vi "Process Mngr.vi"(0 "State In":T5, 1 "Mngr Action":T12, 2 "FP":T11, 7 "Cartridges":T4, 9 "Manual Input":dbl format="%#_13g", 11 "error in (no error)":errorcluster, 12 "Config":T1={"Syringe size"=0, "Syringe address"=0, "# of ports"=0, "Init String"="Z0N1R", "Full Stroke (cnts)"=0, "Model"=enum."XC", "TW Position"=0.0, "Load Position"=0.0, "Bottom Position"=0.0, "Station ID"="", "Default Protocol"=path "", "Dry Time(s)"=0.0, "Python Version"="", "NFC SN Array"=["21121521200223", "21121521200186", "21121521200213", "52541737200062"], "Timing"={"Checking pres and leak"=0.0, "Priming input lines"=0.0, "Rinsing syringe"=0.0, "Filling well X w/ X"=0.0, "Drain well X"=0.0, "Clearing wells and lines"=0.0, "Draining wells"=0.0, "Rinsing all wells"=0.0, "Testing for leaks/clogs"=0.0, "Rinsing wells"=0.0}, "Pressure Specs"={"Pressure max"=0.0, "Pressure min"=0.0, "Decay delta"=0.0, "Pressure time"=0.0, "Conf. R"=0.0, "LeakRateMax"=0.0}}) -> (6 "State Out":T5, 15 "error out":errorcluster)   [LabVIEW 2020]
uses:
  Process Mngr.ctl
  Main Refs.ctl
  Hardware/Tecan/Pump Config.ctl
  Timing Specs.ctl
  Vacuum Specs.ctl
  Cartridges.ctl
  Cartridge Status.ctl
  Commands.ctl
  Lib/Time/Wells.ctl
  Lib/Time/Bottles.ctl
  Process State.ctl
  Vacuum Test.ctl
  Wash Step.ctl
  Results.ctl
  Vacuum Output.ctl
  Cartridge #.ctl
  status update.ctl
  Cartridge Mngr.ctl
  Time elapsed.ctl
  Hardware/DAQ Mngr.ctl
  Hardware/Mot Stage Mngr.ctl
  Update Single Cart.ctl
  Hardware/Denkovi Mngr.ctl
  Hardware/Tricon Mngr.ctl
  Hardware/Tecan/Pump Control.ctl
  Pump Port.ctl
  Hardware/Tecan/Velocity Units.ctl
  Main Globals.vi
  Lib/Utilities.lvlib
panel:
  out "Reports":T6[](array[typedef])
  in  "Pressure Specs":T9
  out "Wash Array":T10[](array[typedef]) {"# of Rinses" max=10}
  # "Tecan Pump"
  # "Pressure"
  # "General"
  # "Timing"
  # "Protocol"
  # "Zaber"
  # "NFC Reader 1"
  # "NFC  Reader 2"
  # "NFC Reader 3"
  # "NFC Reader 4"
  # "Tecan Pump"
  # "Pressure"
  # "General"
  # "Timing"
  # "Protocol"
  # "Zaber"
  # "NFC Reader 1"
  # "NFC  Reader 2"
  # "NFC Reader 3"
  # "NFC Reader 4"
  # "System"
  # "Cartridge Utitlies"
  # "Wells"
  # "times"
  # "from"
  # "State Machine"
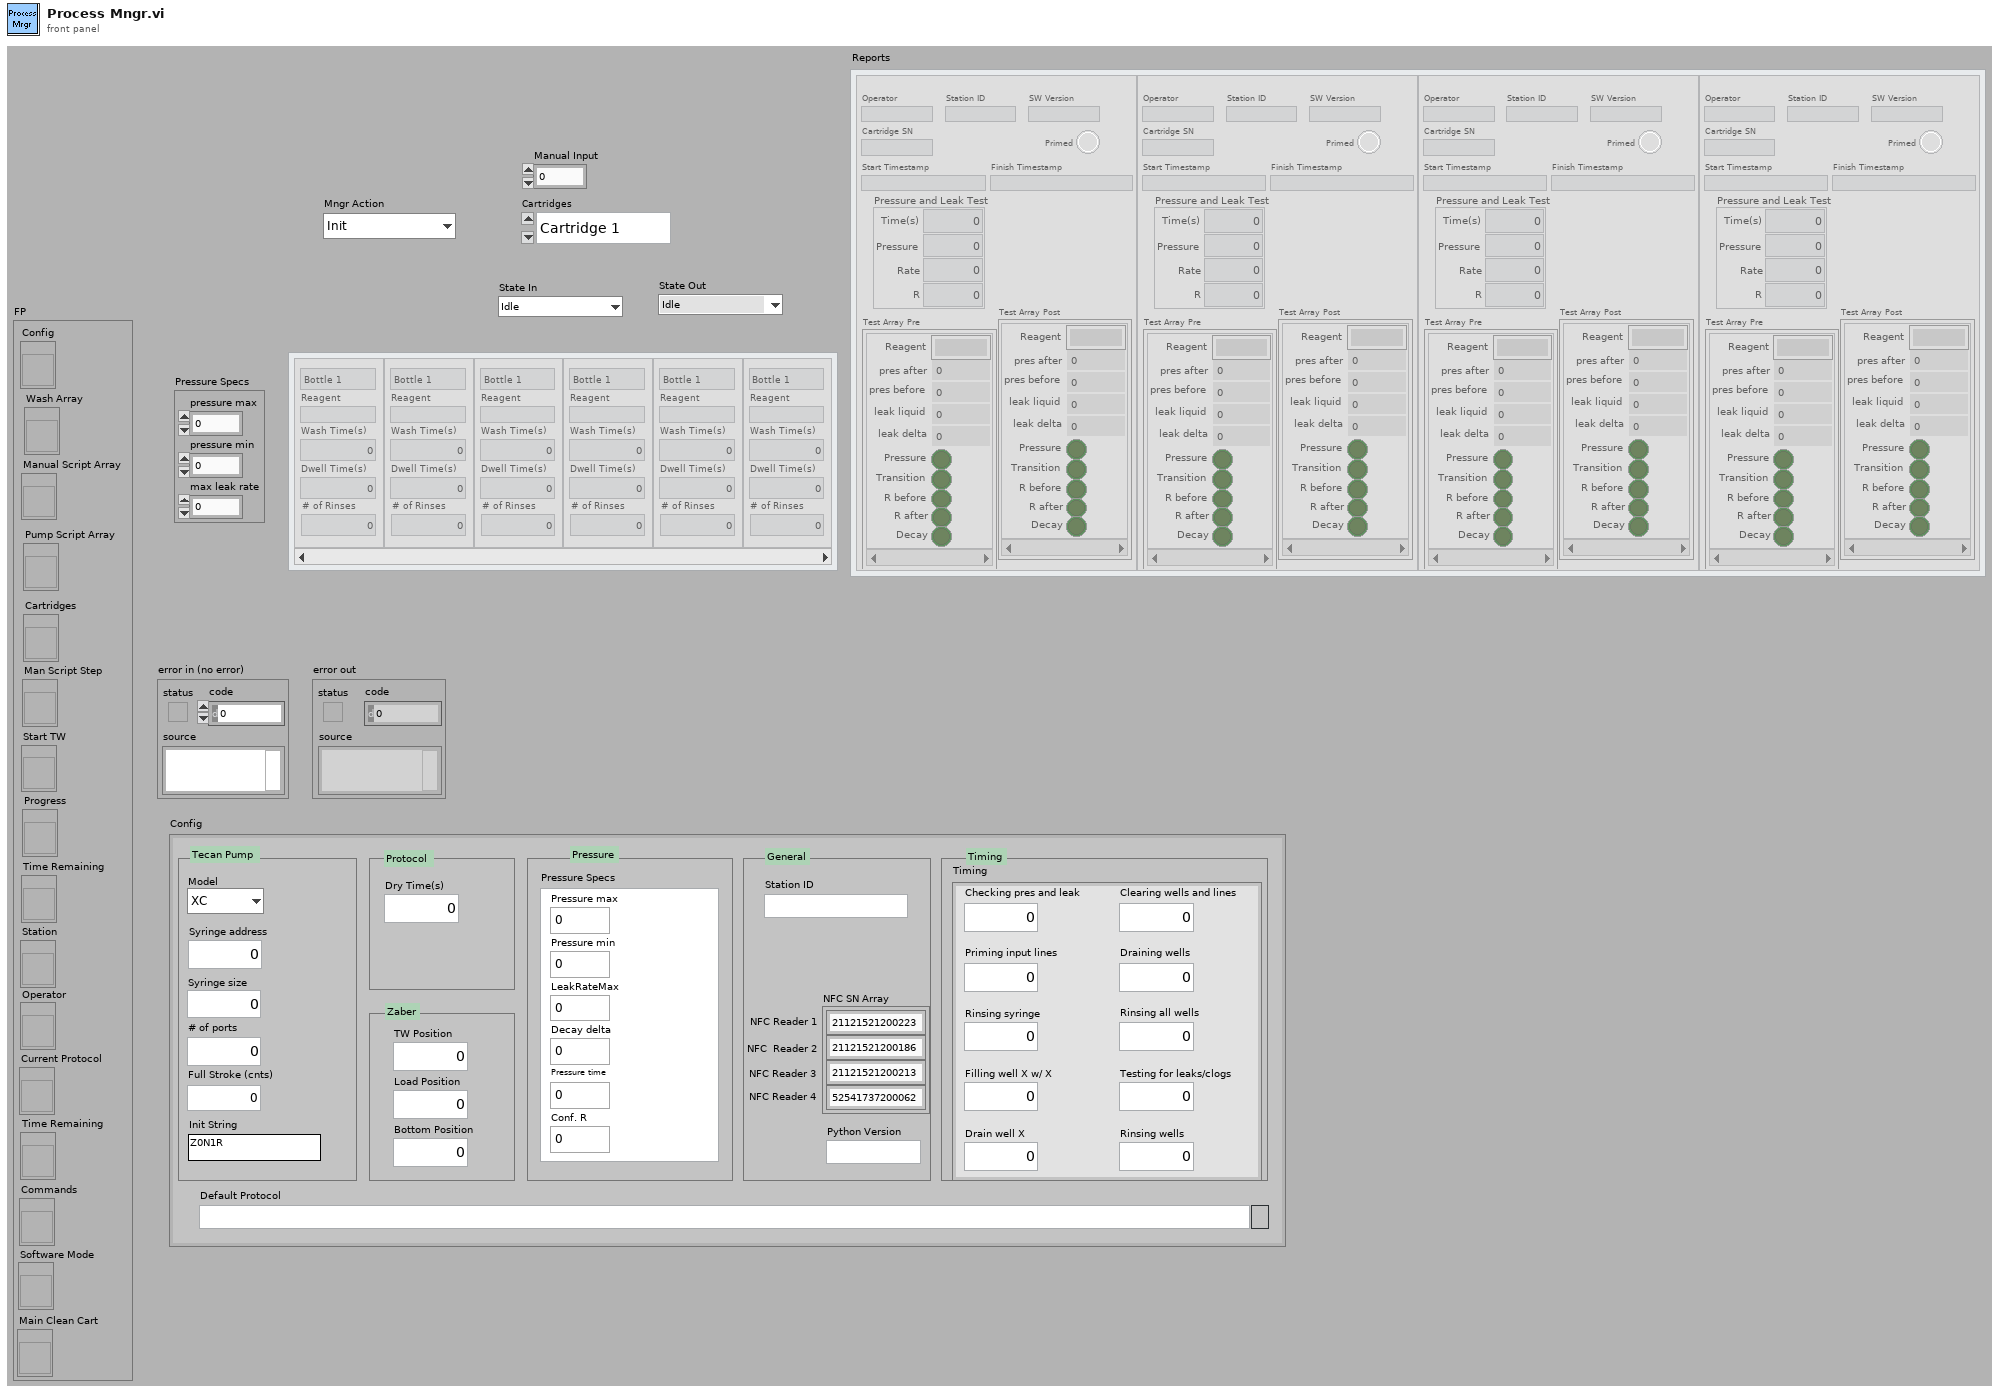
[diagram p1: front panel]
types:
  T1 = typedef "Pump Config.ctl" = cluster{"Syringe size":u32, "Syringe address":u32, "# of ports":u32, "Init String":string, "Full Stroke (cnts)":i32, "Model":enum16{"XC", "Centris"}, "TW Position":dbl, "Load Position":dbl, "Bottom Position":dbl, "Station ID":string, "Default Protocol":path, "Dry Time(s)":dbl, "Python Version":string, "NFC SN Array":string[], "Timing":T2, "Pressure Specs":T3}
  T2 = typedef "Timing Specs.ctl" = cluster{"Checking pres and leak":dbl, "Priming input lines":dbl, "Rinsing syringe":dbl, "Filling well X w/ X":dbl, "Drain well X":dbl, "Clearing wells and lines":dbl, "Draining wells":dbl, "Rinsing all wells":dbl, "Testing for leaks/clogs":dbl, "Rinsing wells":dbl}
  T3 = typedef "Vacuum Specs.ctl" = cluster{"Pressure max":dbl, "Pressure min":dbl, "Decay delta":dbl, "Pressure time":dbl, "Conf. R":dbl, "LeakRateMax":dbl}
  T4 = typedef "Cartridge #.ctl" = enum16{"Cartridge 1", "Cartridge 2", "Cartridge 3", "Cartridge 4"}
  T5 = typedef "Process State.ctl" = enum16{"Idle", "Init", "Check for SN", "Start TW", "SystemLeakTest", "Prime System", "Rinse Wells", "Fill Wells", "PrePresTest", "Apply Pressure", "PostPresTest", "Drain&Rinse", "Dry", "Report", "Finish", "Abort", "Error", "-rinse wells", "-check cartridge", "-clean cartridge", "-drain all", "-fill well"}
  T6 = typedef "Results.ctl" = cluster{"Operator":string, "Station ID":string, "SW Version":string, "Cartridge SN":string, "Primed":bool, "Start Timestamp":string, "Finish Timestamp":string, "Test Array Pre":T7[], "Test Array Post":T7[], "Pressure and Leak Test":T8}
  T7 = typedef "Vacuum Test.ctl" = cluster{"pres after":dbl, "pres before":dbl, "leak liquid":dbl, "leak delta":dbl, "Transition":bool, "Pressure":bool, "R before":bool, "R after":bool, "Reagent":string, "Decay":bool}
  T8 = typedef "Vacuum Output.ctl" = cluster{"Time(s)":dbl, "Pressure":dbl, "Rate":dbl, "R":dbl}
  T9 = cluster{"pressure max":dbl, "pressure min":dbl, "max leak rate":dbl}
  T10 = typedef "Wash Step.ctl" = cluster{"Reagent":string, "Bottle":enum16{"Bottle 1", "Bottle 2", "Bottle 3", "Bottle 4"}, "Wash Time(s)":dbl, "Dwell Time(s)":dbl, "# of Rinses":i16}
  T11 = typedef "Main Refs.ctl" = cluster{"Config":refnum<vi>, "Wash Array":refnum<vi>, "Manual Script Array":refnum<vi>, "Pump Script Array":refnum<vi>, "Cartridges":refnum<vi>, "Man Script Step":refnum<vi>, "Start TW":refnum<vi>, "Progress":refnum<vi>, "Time Remaining":refnum<vi>, "Station":refnum<vi>, "Operator":refnum<vi>, "Current Protocol":refnum<vi>, "Time Remaining":refnum<vi>, "Commands":refnum<vi>, "Software Mode":refnum<vi>, "Main Clean Cart":refnum<vi>}
  T12 = typedef "Process Mngr.ctl" = enum16{"Init", "Run Step", "Update"}
  T13 = enum8{"Enabled", "Disabled", "Disabled and Grayed Out"}
  T14 = typedef "status update.ctl" = enum16{"Cartridge", "Main Status", "Reagent"}
  T15 = typedef "Cartridge Mngr.ctl" = enum16{"Init", "Update", "Detect", "Lock", "Read SN", "Unlock", "Error"}
  T16 = typedef "DAQ Mngr.ctl" = enum16{"Init", "Read Pressure", "Analyze Pressure", "Read Cartridges", "Lock Cartridge", "Unlock Cartridge", "Read PS", "Pinch Valve Engage", "Pinch Valve Disengage", "Close"}
  T17 = typedef "Time elapsed.ctl" = enum16{"Start", "Update", "Read"}
  T18 = typedef "Bottles.ctl" = enum16{"Bottle 1", "Bottle 2", "Bottle 3", "H2O", "Waste"}
  T19 = typedef "Mot Stage Mngr.ctl" = enum16{"Connect", "Init", "Status", "Send Cmd", "Current Pos", "Set Accel", "Set Max Vel", "Home", "Rel Move", "Abs Move", "Close"}
  T20 = typedef "Update Single Cart.ctl" = enum16{"Cart Status", "Cart Reagent"}
  T21 = typedef "Denkovi Mngr.ctl" = enum16{"Search", "Init", "Set Peristaltic", "Set Pressure", "Pres ON", "Vent&Close", "Set All Relays", "Set One Relay", "Read Relays", "Close"}
  T22 = typedef "Pump Control.ctl" = cluster{"Syringe Pos":u32, "Rate":dbl, "Volume":dbl, "Valve":T23, "Action":enum32{"Withdraw", "Dispense", "Stop"}, "Move Type":enum32{"Abs", "Rel"}, "Init":bool, "Empty Syr.":bool, "Full Fill":bool, "Units":T24}
  T23 = typedef "Pump Port.ctl" = enum16{"Bottle 1", "Bottle 2", "Bottle 3", "Bottle 4", "Waste", "Well 1", "Well 2", "Well 3", "Well 4", "Bottle X", "Well X"}
  T24 = typedef "Velocity Units.ctl" = enum16{"ul/s", "ul/min"}
  T25 = typedef "Tricon Mngr.ctl" = enum16{"Init COM", "Set Config", "Init Pump", "Home", "Cmd", "Start Pump", "Set Valve", "Dispense", "Withdraw", "Status", "Close"}
  T26 = typedef "Cartridges.ctl" = cluster{"Cartridge 1":T27, "Cartridge 2":T27, "Cartridge 3":T27, "Cartridge 4":T27, "Current Status":string}
  T27 = typedef "Cartridge Status.ctl" = cluster{"Serial Number":string, "Reagent":string, "Cart Status":string, "Inserted":bool, "Eject":bool}
  T28 = enum16{"Bottle 1", "Bottle 2", "Bottle 3", "Bottle 4"}
  T29 = typedef "Commands.ctl" = cluster{"Drain All Wells":bool, "Rinse All Wells":bool, "Prime":bool, "Well #":T30, "Bottle #":T18, "Fill":bool, "Run State":bool, "State":T5, "Empty Lines":bool, "Clean&Dry Cartridge":bool, "Check for leaks":bool, "Cart Test Array":T7[], "Number of rinses":dbl}
  T30 = typedef "Wells.ctl" = enum16{"Well 1", "Well 2", "Well 3", "Well 4"}
  T31 = cluster{"negative limit switch":bool, "positive limit switch":bool, "home switch":bool, "position marker":bool, "device enable":bool, "quick stop":bool, "general purpose J":bool, "general purpose I":bool, "general purpose H":bool, "general purpose G":bool, "general purpose F":bool, "general purpose E":bool, "general purpose D":bool, "general purpose C":bool, "general purpose B":bool, "general purpose A":bool}
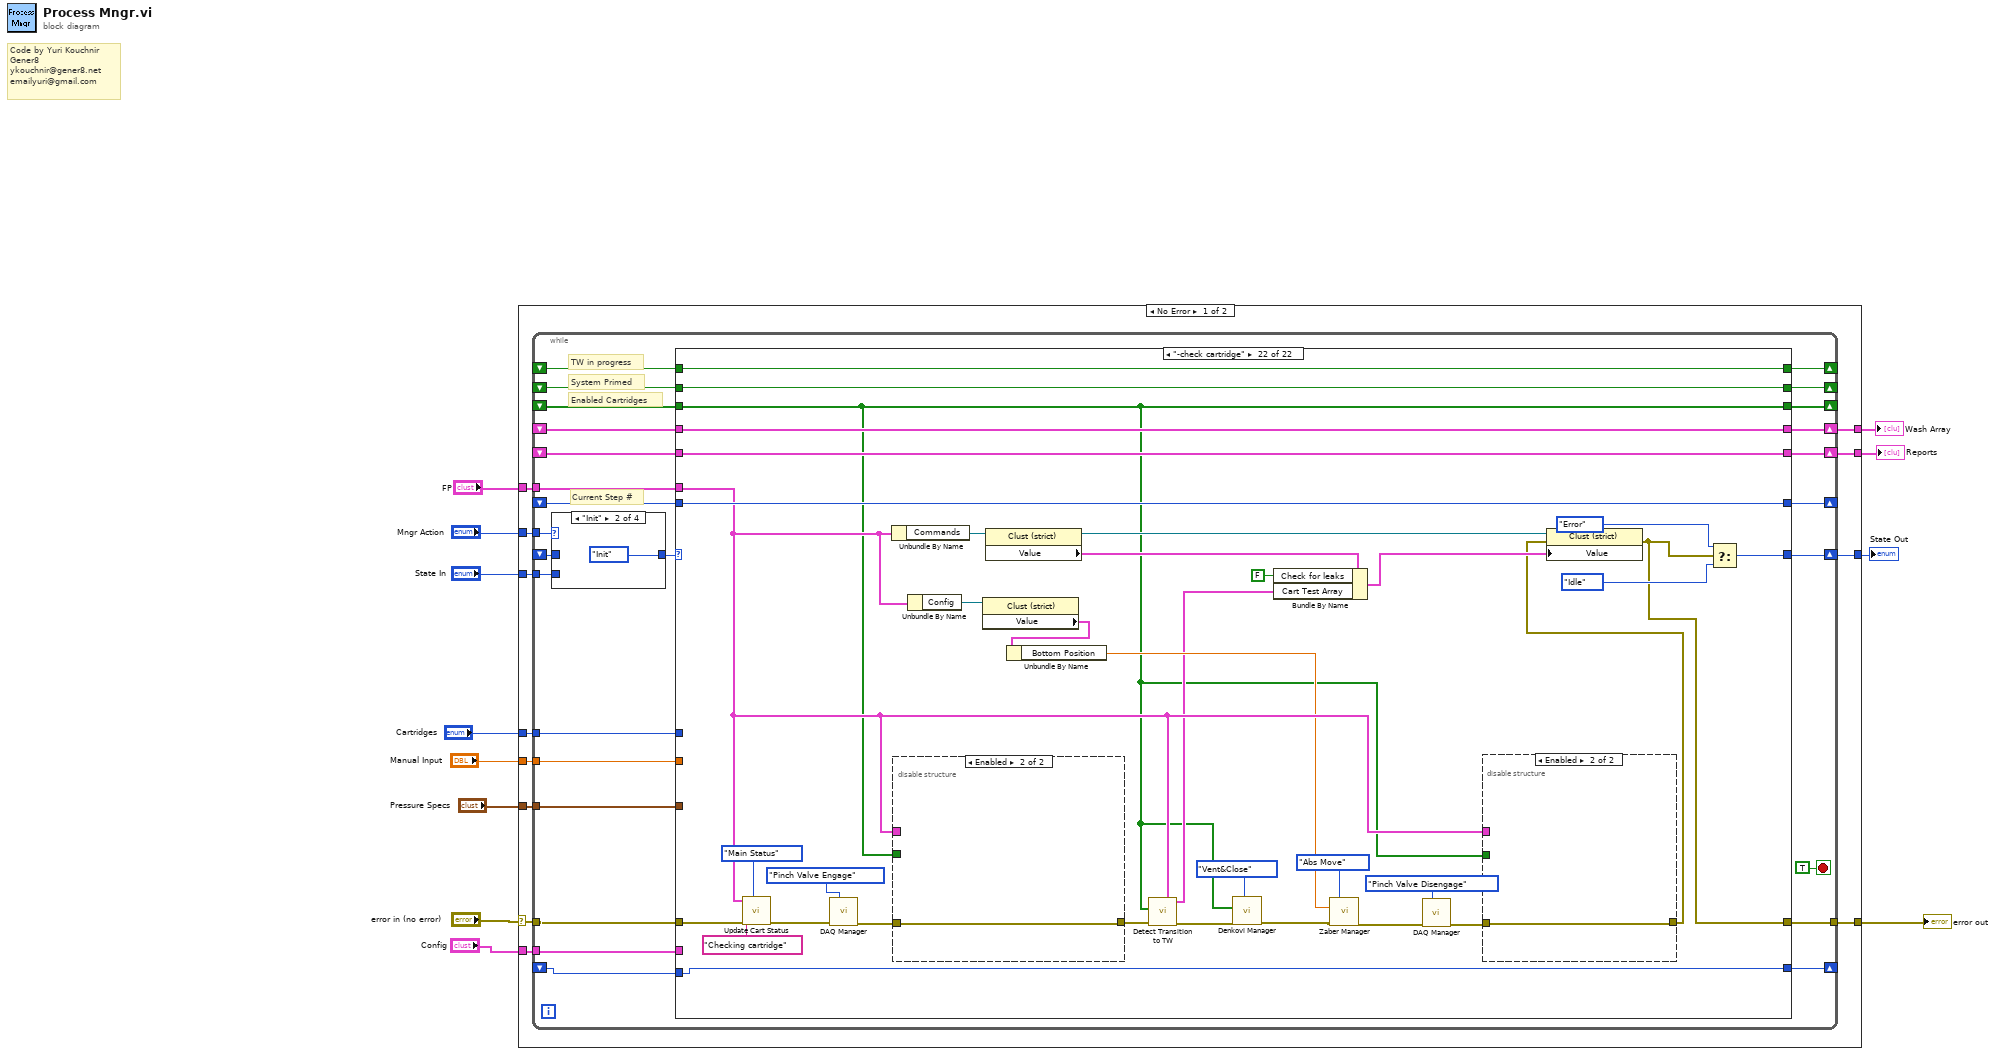
[diagram p0: block diagram]
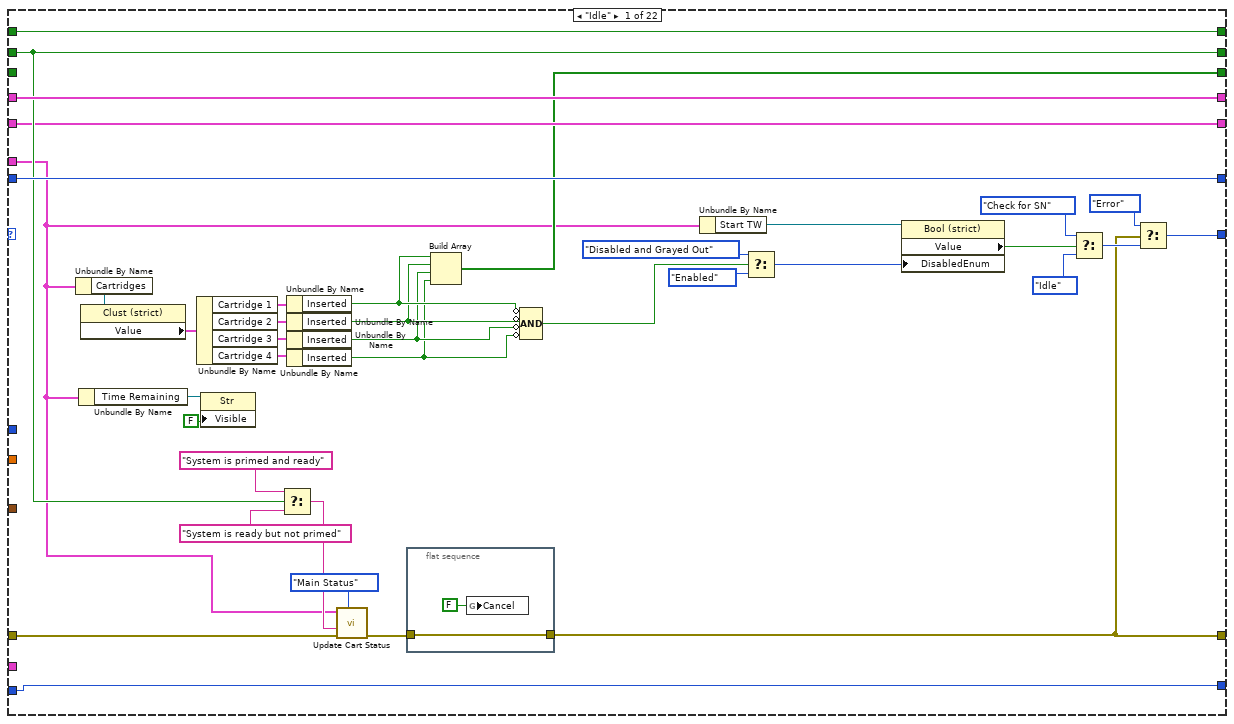
[diagram p5: hidden frame]
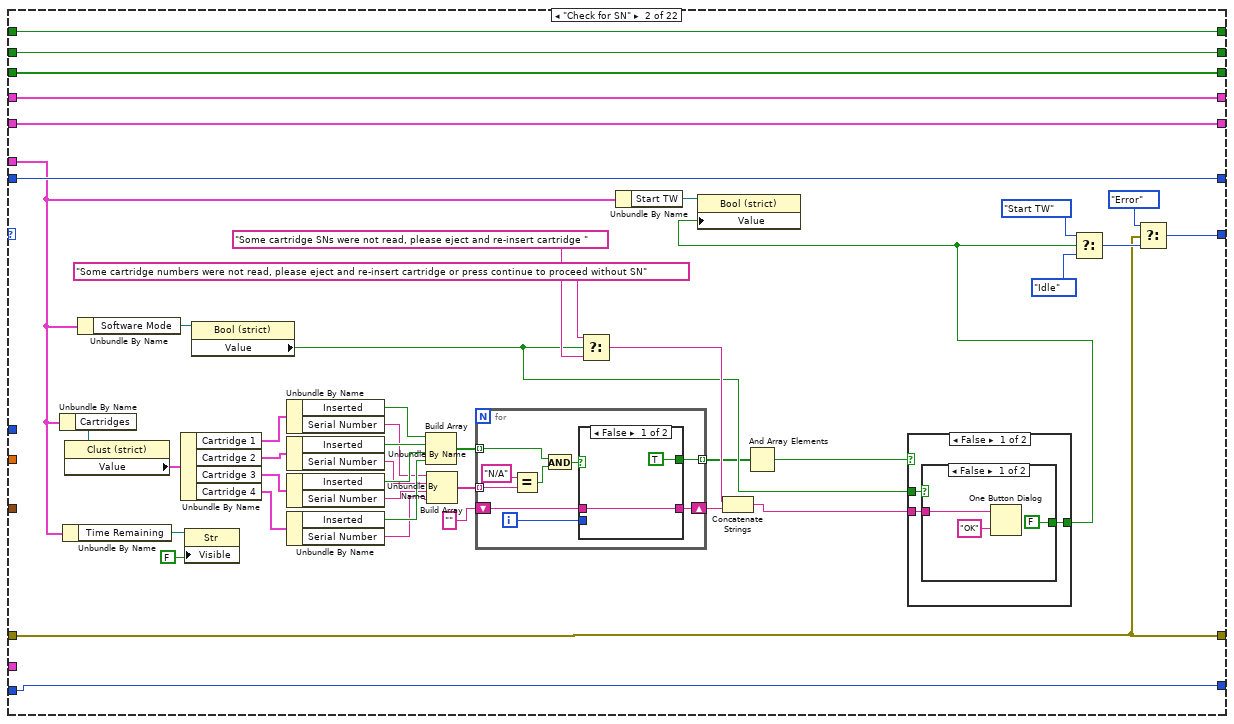
[diagram p6: hidden frame]
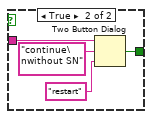
[diagram p7: hidden frame]
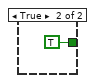
[diagram p8: hidden frame]
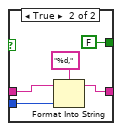
[diagram p9: hidden frame]
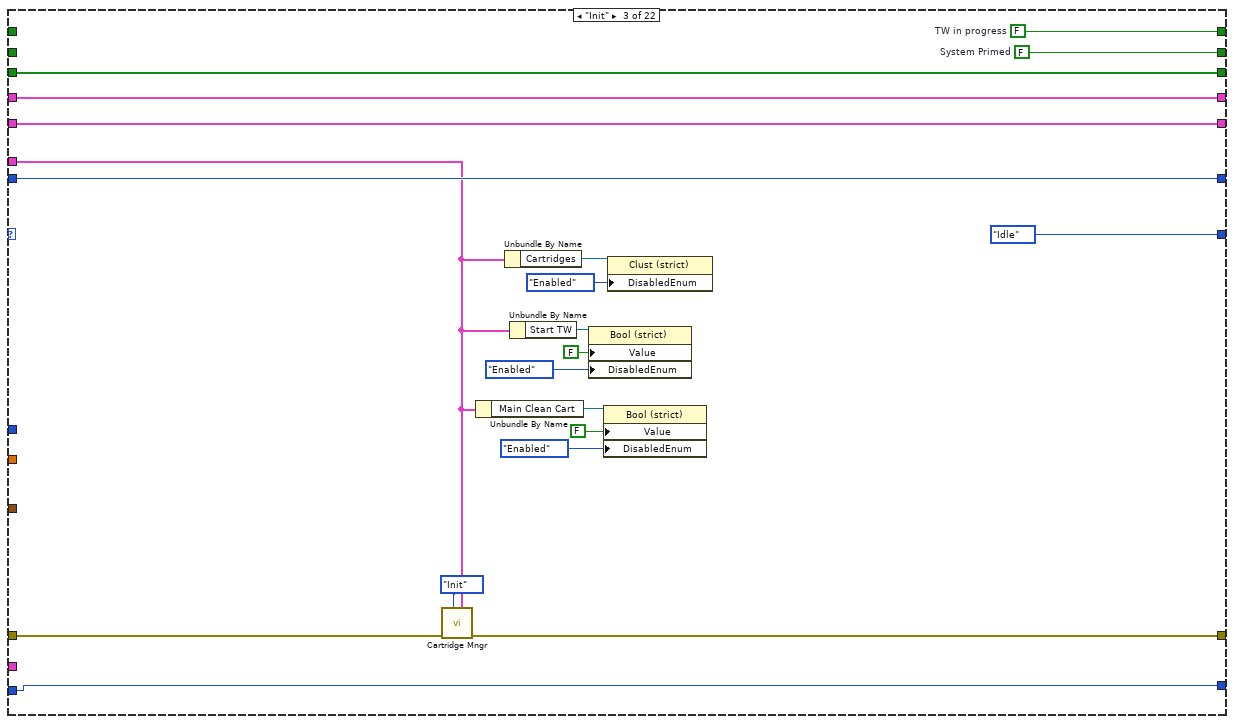
[diagram p10: hidden frame]
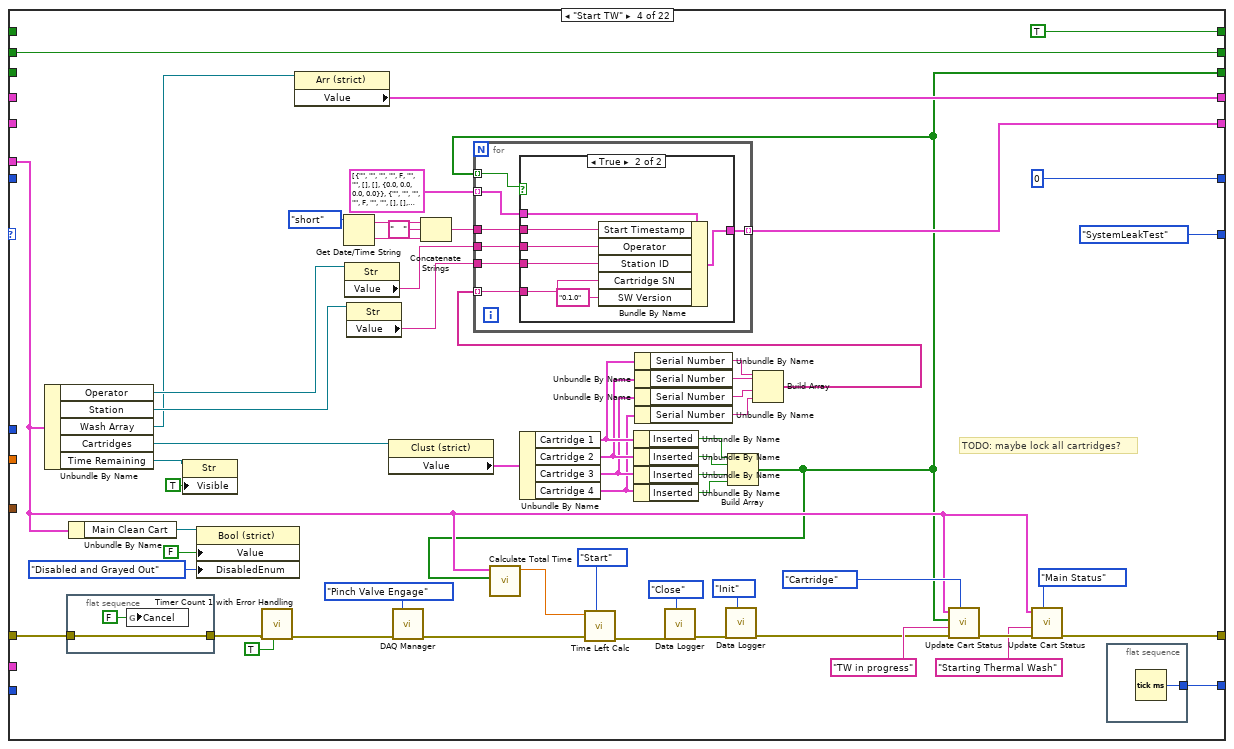
[diagram p11: hidden frame]
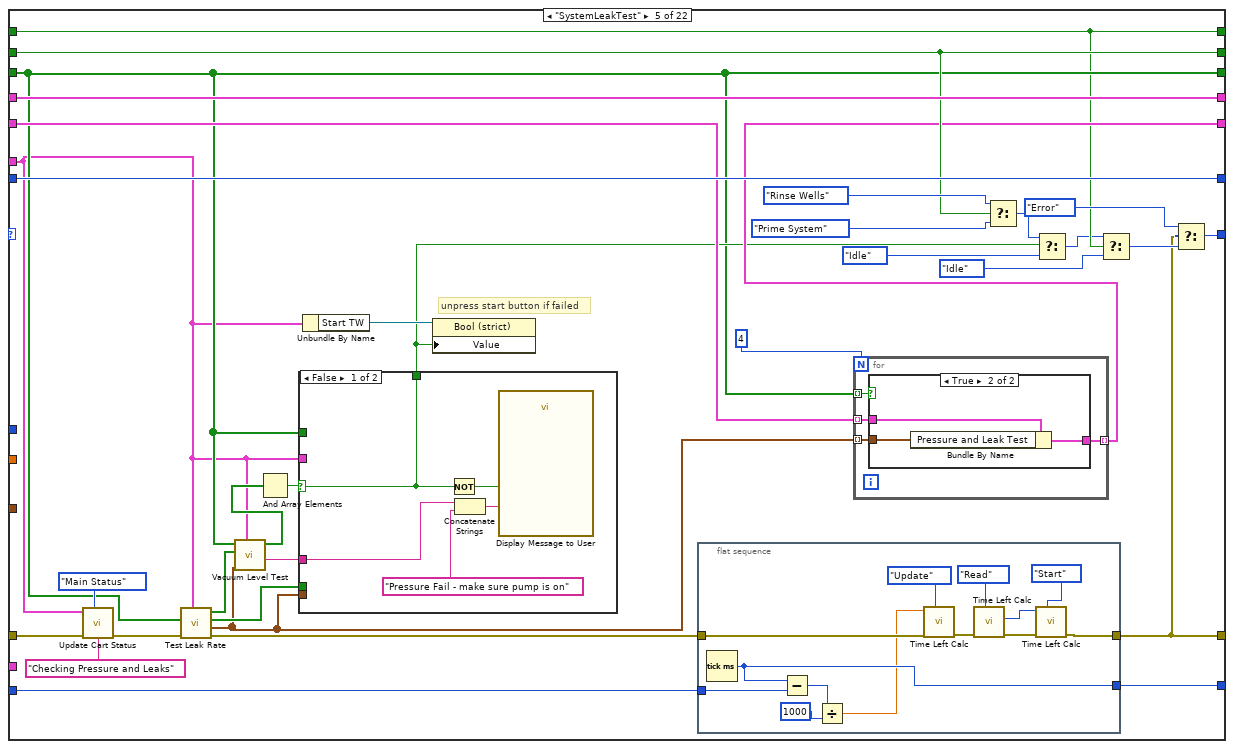
[diagram p13: hidden frame]
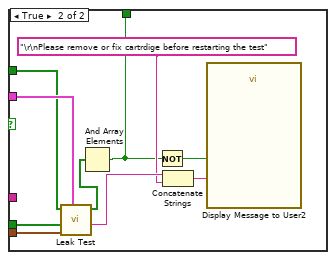
[diagram p14: hidden frame]
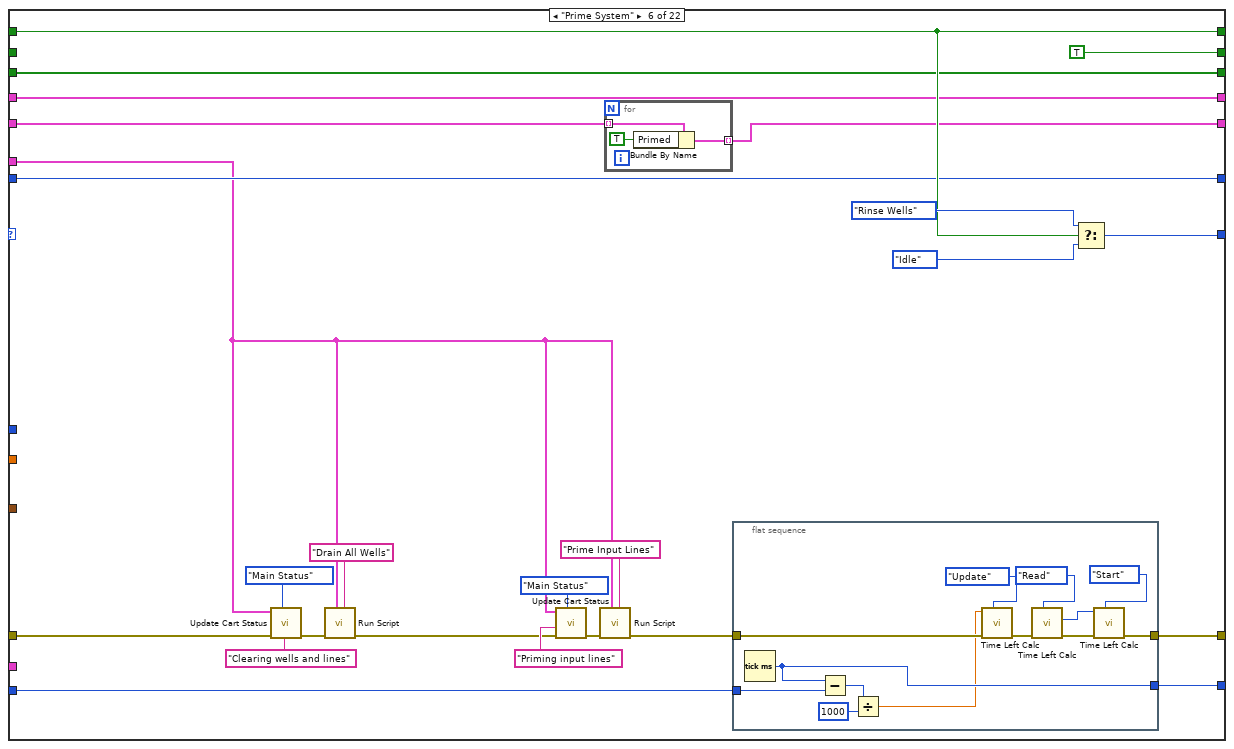
[diagram p16: hidden frame]
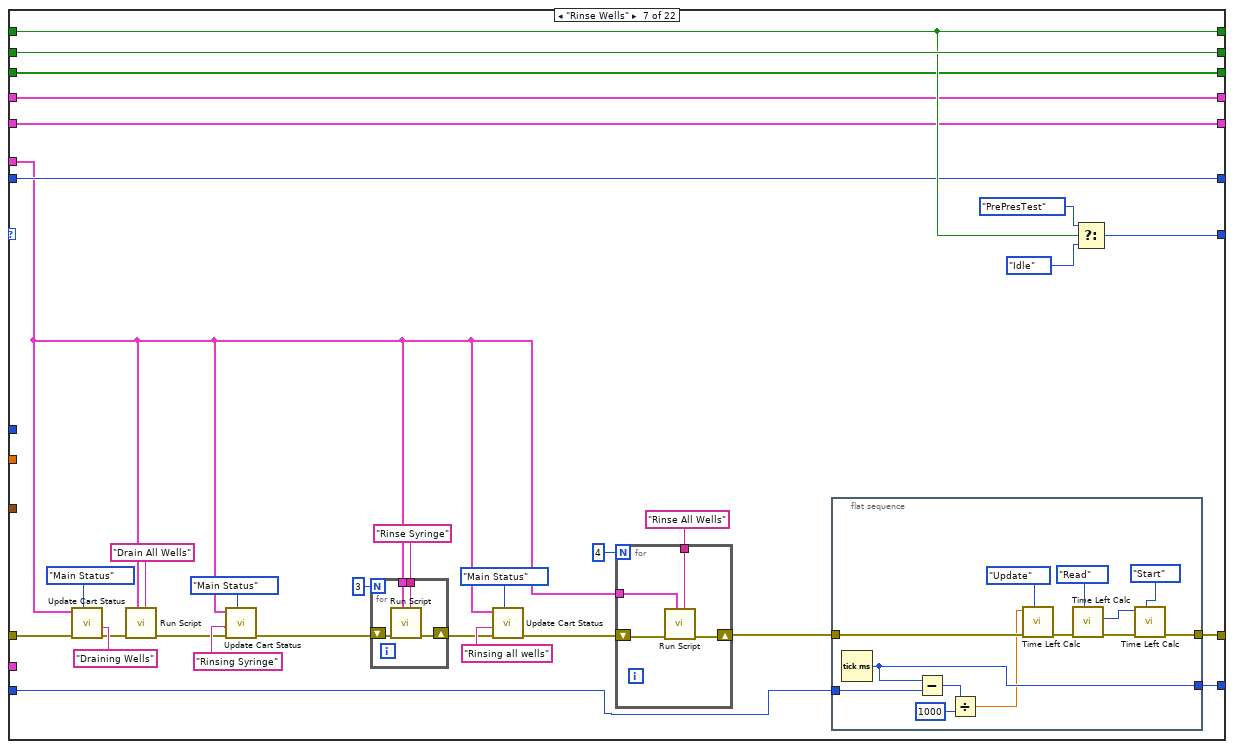
[diagram p17: hidden frame]
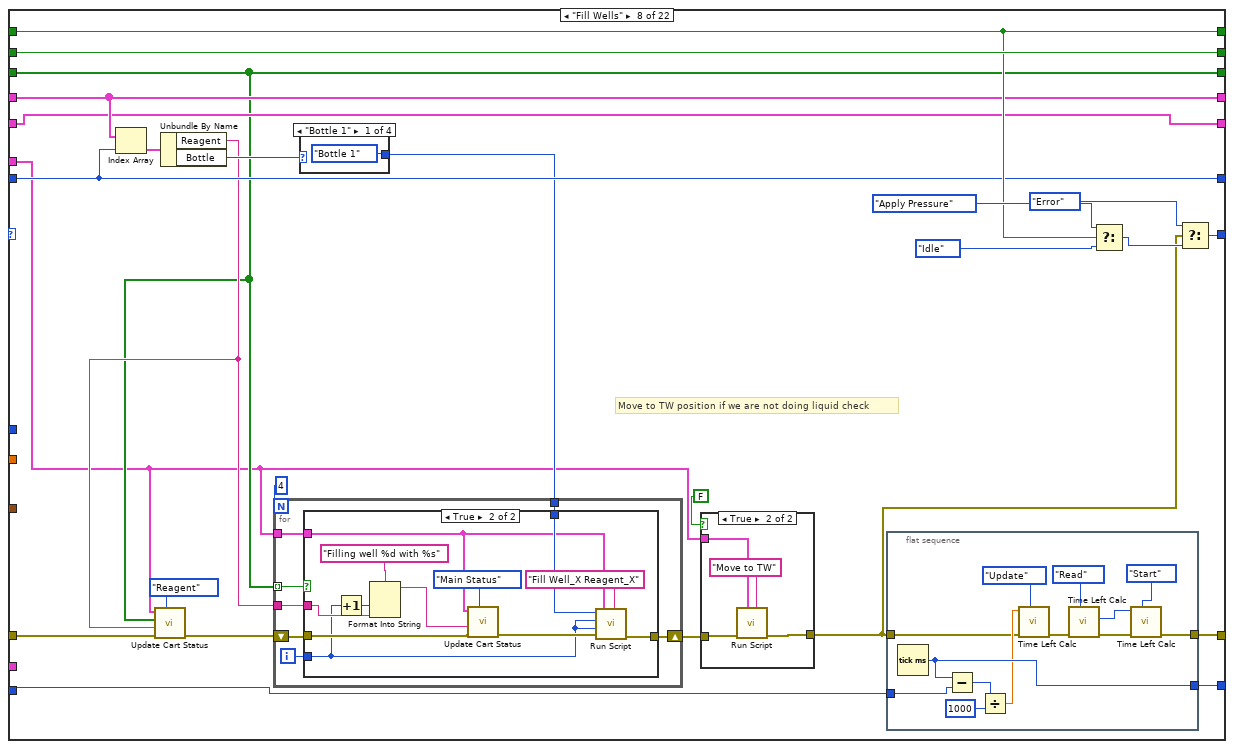
[diagram p18: hidden frame]
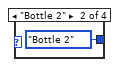
[diagram p20: hidden frame]
diagram:
  # "Code by Yuri Kouchnir\nGener8\nykouchnir@gener8.net\nemailyuri@gmail.com"
  n1 = case shown="No Error" "error in (no error)" {
    selector: "error in (no error)" -> [w24 w1274]
    tunnel: [w23 w1274] -> w11
    tunnel: "Mngr Action" -> [w22 _]
    tunnel: "FP" -> [w21 _]
    tunnel: "Pressure Specs" -> [w20 _]
    tunnel: [w19 _] -> w7
    tunnel: [w18 _] -> w6
    tunnel: [w17 _] -> w4
    tunnel: "State In" -> [w16 _]
    tunnel: "Cartridges" -> [w15 _]
    tunnel: "Manual Input" -> [w14 _]
    tunnel: "Config" -> [w13 _]
    frame No Error {
      n2 = while {
        tunnel: w24 -> [w50]
        tunnel: [w49] -> w23
        tunnel: w22 -> [w44]
        shift-right: [w48] -> w19
        shift-left: _ -> [w46]
        tunnel: w21 -> [w47]
        shift-right: [w43] -> _
        shift-left: _ -> [w42]
        shift-right: [w41] -> w18
        shift-left: _ -> [w40]
        shift-right: [w39] -> _
        shift-left: _ -> [w38]
        shift-right: [w37] -> _
        shift-left: _ -> [w36]
        shift-right: [w35] -> _
        shift-left: _ -> [w34]
        tunnel: w20 -> [w33]
        shift-right: [w32] -> w17
        shift-left: _ -> [w31]
        tunnel: w16 -> [w30]
        tunnel: w15 -> [w29]
        tunnel: w14 -> [w28]
        shift-right: [w27] -> _
        shift-left: _ -> [w26]
        tunnel: w13 -> [w25]
        stop <- TRUE stop-if-true
        # "Current Step #"
        # "Enabled Cartridges"
        # "System Primed"
        # "TW in progress"
        n3 = case shown="\"Init\"" w44 {
          tunnel: w46 -> [w52 _ _ w55]
          tunnel: [w52 Process_State."Init" ("State") w54 w55] -> w45
          tunnel: w30 -> [_ _ w54 _]
          frame Default {
          }
          frame "Init" {
          }
          frame "Run Step" {
          }
          frame "Update" {
          }
        }
        n4 = case shown="\"-check cartridge\"" w45 {
          tunnel: w50 -> [w63 w104 w167 w213 w294 w337 w394 w434 w515 w599 w669 w749 w866 w915 w950 w966 w1032 w1050 w1083 w1106 w1161 w1234]
          tunnel: [w61 w104 w180 w234 w267 w340 w376 w429 w498 w587 w658 w741 w854 w914 w941 w969 w1024 w1041 w1075 w1100 w1145 w1216] -> w49
          tunnel: [w84 w131 Process_State."Idle" ("State") Process_State."SystemLeakTest" ("State") w291 w357 w404 w444 w518 w614 w672 w771 w874 Process_State."Idle" ("State") Process_State."Idle" ("State") Process_State."Finish" ("State") Process_State."Idle" ("State") w1060 w1091 w1114 w1164 w1237] -> w48
          tunnel: w47 -> [w58 w106 w169 w192 w268 w342 w378 w430 w506 w594 w661 w750 w858 w918 w938 w964 w1015 w1043 w1086 w1109 w1122 w1221]
          tunnel: [w82 w130 w185 w211 w289 TRUE ("System Primed") w401 w449 w521 w618 w675 w776 w886 w931 w960 w980 w1038 w1062 w1095 w1118 w1151 w1223] -> w43
          tunnel: w42 -> [w82 w130 _ w211 w289 _ w401 w449 w521 w618 w675 w776 w886 w931 w960 w980 w1038 w1062 w1095 w1118 w1151 w1223]
          tunnel: [w91 w137 w181 w199 w296 w351 w397 w439 w517 w605 w671 w767 w873 w930 w959 w979 w1037 w1059 w1089 w1112 w1163 w1236] -> w41
          tunnel: w40 -> [w91 w137 w181 _ w296 w351 w397 w439 w517 w605 w671 w767 w873 w930 w959 w979 w1037 w1059 w1089 w1112 w1163 w1236]
          tunnel: [w93 w139 w184 TRUE ("TW in progress") w272 w354 w400 w447 w503 w617 w656 w745 w869 w929 FALSE ("TW in progress") w978 FALSE ("TW in progress") w1047 w1094 w1117 w1157 w1230] -> w39
          tunnel: w38 -> [w93 w139 _ _ w272 w354 w400 w447 w503 w617 w656 w745 w869 w929 _ w978 _ w1047 w1094 w1117 w1157 w1230]
          tunnel: [w92 w138 w182 0 w295 w352 w398 w443 w511 w611 w665 w768 w870 w928 w958 w977 w1036 w1046 w1090 w1113 w1158 w1231] -> w37
          tunnel: w36 -> [w92 w138 w182 _ w295 w352 w398 w443 w511 w611 w665 w769 w870 w928 w958 w977 w1036 w1046 w1090 w1113 w1158 w1231]
          tunnel: [w64 w116 w183 w191 w273 w353 w399 w432 w505 w593 w660 w755 w857 w927 w957 w962 w1033 w1040 w1087 w1110 w1125 w1211] -> w35
          tunnel: w34 -> [_ w116 w183 _ w273 w353 w399 w432 w502 w593 w647 w755 w857 w927 w957 w962 w1033 w1040 w1087 w1110 w1125 w1211]
          tunnel: w33 -> [_ _ _ _ _ _ _ _ _ w607 _ _ w881 _ _ _ _ _ _ _ _ _]
          tunnel: [w78 w129 w173 w227 w281 w347 w380 w437 w509 w602 w663 w765 w868 w917 w956 w968 w1022 w1058 w1088 w1111 w1123 w1215] -> w32
          tunnel: w31 -> [w78 w129 w173 _ w283 w348 w380 w437 w510 w602 w664 w765 w868 w917 w956 w970 w1022 w1058 w1088 w1111 w1123 w1215]
          tunnel: w29 -> [_ _ _ _ _ _ _ _ _ _ _ _ _ _ _ _ _ _ _ _ _ _]
          tunnel: w28 -> [_ _ _ _ _ _ _ _ _ _ _ _ _ _ _ _ _ w1045 _ _ _ _]
          tunnel: [w56 w96 w168 w190 w264 w338 w374 w428 w495 w586 w649 w740 w852 w913 w940 w961 w1014 w1039 w1074 w1098 w1121 w1209] -> w27
          tunnel: w26 -> [w56 w96 w168 _ w266 w341 w377 w426 w494 _ w648 w739 _ w913 w940 w961 w1014 w1039 w1074 w1098 w1121 w1209]
          tunnel: w25 -> [_ _ _ _ _ _ _ _ _ _ _ _ _ _ w937 _ _ _ _ _ _ _]
          frame "Idle" {
            n5 = Unbundle By Name(w58) -> ("Cartridges"=w73:refnum<vi>)
            n6 = Unbundle By Name(w58) -> ("Time Remaining"=w60:refnum<vi>)
            n7 = property class="Clust (strict)"(reference=w73) -> ("Value"=w77:T26)  [unwired: 1 in, 2 out]
            n8 = Unbundle By Name(w77) -> ("Cartridge 1"=w72:T27, "Cartridge 2"=w76:T27, "Cartridge 3"=w75:T27, "Cartridge 4"=w74:T27)
            n9 = property class="Str"(reference=w60, "Visible"=FALSE) -> ()  [unwired: 1 in, 2 out]
            n10 = Select(t="System is primed and ready" ("Reagent"), s=w82, f="System is ready but not primed" ("Reagent")) -> (s? t:f=w79:string)
            n11 = Unbundle By Name(w72) -> ("Inserted"=w68:bool)
            n12 = Unbundle By Name(w76) -> ("Inserted"=w67:bool)
            n13 = Unbundle By Name(w75) -> ("Inserted"=w66:bool)
            n14 = Unbundle By Name(w74) -> ("Inserted"=w65:bool)
            n15 = call "Update Cart Status.vi"("Selection"=status_update."Main Status", "error in (no error)"=w63, "String"=w79, "FP"=w58) -> ("error out"=w62:errorcluster)  [unwired: 7 in]
            n16 = flat-sequence {
              tunnel: w62 -> [w95]
              tunnel: [w95] -> w61
              frame #0 {
                n17 = global write "Main Globals.vi" "Cancel"(FALSE ("Cancel")) -> ()
              }
            }
            n18 = Build Array(w68, w67, w66, w65) -> (w64:bool[])
            n19 = Compound Arithmetic op=AND(invert w68, invert w67, invert w66, invert w65) -> (w57:bool)
            n20 = Unbundle By Name(w58) -> ("Start TW"=w90:refnum<vi>)
            n21 = Select(t=T13."Disabled and Grayed Out" ("Disabled"), s=w57, f=T13."Enabled" ("Disabled")) -> (s? t:f=w69:T13)
            n22 = property class="Bool (strict)"(reference=w90, "DisabledEnum"=w69) -> ("Value"=w89:bool)  [unwired: 1 in, 2 out]
            n23 = Select(t=Process_State."Check for SN" ("State"), s=w89, f=Process_State."Idle" ("State")) -> (s? t:f=w86:T5)
            n24 = Select(t=Process_State."Error" ("State"), s=w61, f=w86) -> (s? t:f=w84:T5)
          }
          frame "Check for SN" {
            n25 = Unbundle By Name(w106) -> ("Cartridges"=w124:refnum<vi>)
            n26 = Unbundle By Name(w106) -> ("Time Remaining"=w118:refnum<vi>)
            n27 = property class="Clust (strict)"(reference=w124) -> ("Value"=w128:T26)  [unwired: 1 in, 2 out]
            n28 = Unbundle By Name(w106) -> ("Software Mode"=w105:refnum<vi>)
            n29 = Unbundle By Name(w128) -> ("Cartridge 1"=w123:T27, "Cartridge 2"=w127:T27, "Cartridge 3"=w126:T27, "Cartridge 4"=w125:T27)
            n30 = property class="Str"(reference=w118, "Visible"=FALSE) -> ()  [unwired: 1 in, 2 out]
            n31 = property class="Bool (strict)"(reference=w105) -> ("Value"=w100:bool)  [unwired: 1 in, 2 out]
            n32 = Unbundle By Name(w123) -> ("Inserted"=w122:bool, "Serial Number"=w115:string)
            n33 = Unbundle By Name(w127) -> ("Inserted"=w121:bool, "Serial Number"=w114:string)
            n34 = Unbundle By Name(w126) -> ("Inserted"=w120:bool, "Serial Number"=w113:string)
            n35 = Unbundle By Name(w125) -> ("Inserted"=w119:bool, "Serial Number"=w112:string)
            n36 = Build Array(w122, w121, w120, w119) -> (w111:bool[])
            n37 = Build Array(w115, w114, w113, w112) -> (w110:string[])
            n38 = for {
              tunnel: w111 -> [w154] mode=indexing
              tunnel: w110 -> [w157] mode=indexing
              shift-right: [w152] -> w107
              shift-left: "" ("Serial Number") -> [w158]
              tunnel: [w151] -> w99 mode=indexing
              i -> [w159]
              n39 = Equal?(x="N/A", y=w157) -> (x = y?=w155:bool)
              n40 = And(x=w154, y=w155) -> (x .and. y?=w153:bool)
              n41 = case shown="False" w153 {
                tunnel: w159 -> [_ w166]
                tunnel: w158 -> [w161 w165]
                tunnel: [w161 w164] -> w152
                tunnel: [TRUE FALSE] -> w151
                frame False {
                }
                frame True {
                  n42 = Format Into String(format string="%d,", initial string=w165, w166) -> (resulting string=w164:string)  [unwired: 1 in, 1 out]
                }
              }
            }
            n43 = Select(t="Some cartridge numbers were not read, please eject and re-insert cartridge or press continue to proceed without SN" ("message"), s=w100, f="Some cartridge SNs were not read, please eject and re-insert cartridge " ("message")) -> (s? t:f=w101:string)
            n44 = Unbundle By Name(w106) -> ("Start TW"=w136:refnum<vi>)
            n45 = Concatenate Strings(w101, w107) -> (w108:string)
            n46 = And Array Elements(Boolean array=w99) -> (logical AND=w98:bool)
            n47 = case shown="False" w98 {
              tunnel: w108 -> [w142 _]
              tunnel: w100 -> [w141 _]
              tunnel: [w140 TRUE ("T button?")] -> w97
              frame False {
                n48 = case shown="False" w141 {
                  tunnel: w142 -> [w144 w149]
                  tunnel: [FALSE ("T button?") w146] -> w140
                  frame False {
                    n49 = One Button Dialog(message=w144, button name ("OK")="OK") -> ()  [unwired: 1 out]
                  }
                  frame True {
                    n50 = Two Button Dialog(message=w149, 1:"restart" ("T button name (\"OK\")"), 2:"continue\nwithout SN" ("T button name (\"OK\")")) -> (T button?=w146:bool)
                  }
                }
              }
              frame True {
              }
            }
            n51 = property class="Bool (strict)"(reference=w136, "Value"=w97) -> ()  [unwired: 1 in, 2 out]
            n52 = Select(t=Process_State."Start TW" ("State"), s=w97, f=Process_State."Idle" ("State")) -> (s? t:f=w133:T5)
            n53 = Select(t=Process_State."Error" ("State"), s=w104, f=w133) -> (s? t:f=w131:T5)
          }
          frame "Init" {
            w184 = FALSE  # TW in progress
            w185 = FALSE  # System Primed
            n54 = call "Cartridge Mngr.vi"("Main References"=w169, "Mngr Action"=Cartridge_Mngr."Init", "error in (no error)"=w167) -> ("error out"=w180:errorcluster)  [unwired: 6 in, 2 out]
            n55 = Unbundle By Name(w169) -> ("Main Clean Cart"=w170:refnum<vi>)
            n56 = Unbundle By Name(w169) -> ("Cartridges"=w178:refnum<vi>)
            n57 = Unbundle By Name(w169) -> ("Start TW"=w176:refnum<vi>)
            n58 = property class="Bool (strict)"(reference=w176, "Value"=FALSE, "DisabledEnum"=T13."Enabled" ("Disabled")) -> ()  [unwired: 1 in, 2 out]
            n59 = property class="Bool (strict)"(reference=w170, "Value"=FALSE, "DisabledEnum"=T13."Enabled" ("Disabled")) -> ()  [unwired: 1 in, 2 out]
            n60 = property class="Clust (strict)"(reference=w178, "DisabledEnum"=T13."Enabled" ("Disabled")) -> ()  [unwired: 1 in, 2 out]
          }
          frame "Start TW" {
            # "TODO: maybe lock all cartridges?"
            n61 = Unbundle By Name(w192) -> ("Operator"=w217:refnum<vi>, "Station"=w215:refnum<vi>, "Wash Array"=w204:refnum<vi>, "Cartridges"=w212:refnum<vi>, "Time Remaining"=w197:refnum<vi>)
            n62 = flat-sequence {
              tunnel: w213 -> [w248]
              tunnel: [w248] -> w208
              frame #0 {
                n63 = global write "Main Globals.vi" "Cancel"(FALSE ("Cancel")) -> ()
              }
            }
            n64 = Unbundle By Name(w192) -> ("Main Clean Cart"=w193:refnum<vi>)
            n65 = property class="Str"(reference=w197, "Visible"=TRUE) -> ()  [unwired: 1 in, 2 out]
            n66 = property class="Bool (strict)"(reference=w193, "Value"=FALSE, "DisabledEnum"=T13."Disabled and Grayed Out" ("Disabled")) -> ()  [unwired: 1 in, 2 out]
            n67 = call "Timer Count 1 with Error Handling.vi"("Reset"=TRUE, "error in (no error)"=w208) -> ("error out"=w188:errorcluster)  [unwired: 6 in, 3 out]
            n68 = property class="Arr (strict)"(reference=w204) -> ("Value"=w199:T10[])  [unwired: 1 in, 2 out]
            n69 = Get Date/Time String(date format (0)=enum16{"short", "long", "abbreviated"}."short") -> (date string=w231:string, time string=w230:string)  [unwired: 2 in]
            n70 = property class="Str"(reference=w217) -> ("Value"=w216:string)  [unwired: 1 in, 2 out]
            n71 = property class="Str"(reference=w215) -> ("Value"=w214:string)  [unwired: 1 in, 2 out]
            n72 = property class="Clust (strict)"(reference=w212) -> ("Value"=w210:T26)  [unwired: 1 in, 2 out]
            n73 = call "DAQ Manager.vi"("DAQ Mngr Action"=DAQ_Mngr."Pinch Valve Engage", "error in (no error)"=w188) -> ("error out"=w187:errorcluster)  [unwired: 7 in, 6 out]
            n74 = Concatenate Strings(w231, "   " ("string"), w230) -> (w228:string)
            n75 = Unbundle By Name(w210) -> ("Cartridge 1"=w226:T27, "Cartridge 2"=w225:T27, "Cartridge 3"=w224:T27, "Cartridge 4"=w223:T27)
            n76 = Unbundle By Name(w226) -> ("Inserted"=w243:bool)
            n77 = Unbundle By Name(w225) -> ("Inserted"=w242:bool)
            n78 = Unbundle By Name(w224) -> ("Inserted"=w241:bool)
            n79 = Unbundle By Name(w223) -> ("Inserted"=w240:bool)
            n80 = Unbundle By Name(w226) -> ("Serial Number"=w222:string)
            n81 = Unbundle By Name(w225) -> ("Serial Number"=w221:string)
            n82 = Unbundle By Name(w224) -> ("Serial Number"=w220:string)
            n83 = Unbundle By Name(w223) -> ("Serial Number"=w219:string)
            n84 = Build Array(w243, w242, w241, w240) -> (w191:bool[])
            n85 = call "Calculate Total Time.vi"("Boolean array"=w191, "FP"=w192) -> ("Total Time(s)"=w198:dbl)  [unwired: 9 in]
            n86 = call "Time Left Calc.vi"("Enum"=Time_elapsed."Start", "error in (no error)"=w187, "Time"=w198) -> ("error out"=w201:errorcluster)  [unwired: 6 in, 2 out]
            n87 = call "Data Logger.vi"("Action"=enum16{"Init", "Save", "Close"}."Close", "error in"=w201) -> ("error out"=w202:errorcluster)  [unwired: 9 in]
            n88 = call "Data Logger.vi"("Action"=enum16{"Init", "Save", "Close"}."Init", "error in"=w202) -> ("error out"=w203:errorcluster)  [unwired: 9 in]
            n89 = Build Array(w222, w221, w220, w219) -> (w218:string[])
            n90 = for {
              tunnel: T6[] [{"Operator"="", "Station ID"="", "SW Version"="", "Cartridge SN"="", "Primed"=FALSE, "Start Timestamp"="", "Finish Timestamp"="", "Test Array Pre"=[], "Test Array Post"=[], "Pressure and Leak Test"={"Time(s)"=0.0, "Pressure"=0.0, "Rate"=0.0, "R"=0.0}}, {"Operator"="", "Station ID"="", "SW Version"="", "Cartridge SN"="", "Primed"=FALSE, "Start Timestamp"="", "Finish Timestamp"="", "Test Array Pre"=[], "Test Array Post"=[], "Pressure and Leak Test"={"Time(s)"=0.0, "Pressure"=0.0, "Rate"=0.0, "R"=0.0}}, {"Operator"="", "Station ID"="", "SW Version"="", "Cartridge SN"="", "Primed"=FALSE, "Start Timestamp"="", "Finish Timestamp"="", "Test Array Pre"=[], "Test Array Post"=[], "Pressure and Leak Test"={"Time(s)"=0.0, "Pressure"=0.0, "Rate"=0.0, "R"=0.0}}, {"Operator"="", "Station ID"="", "SW Version"="", "Cartridge SN"="", "Primed"=FALSE, "Start Timestamp"="", "Finish Timestamp"="", "Test Array Pre"=[], "Test Array Post"=[], "Pressure and Leak Test"={"Time(s)"=0.0, "Pressure"=0.0, "Rate"=0.0, "R"=0.0}}] ("Reports") -> [w255] mode=indexing
              tunnel: w228 -> [w254]
              tunnel: [w253] -> w227 mode=indexing
              tunnel: w191 -> [w252] mode=indexing
              tunnel: w218 -> [w251] mode=indexing
              tunnel: w216 -> [w250]
              tunnel: w214 -> [w249]
              n91 = case shown="True" w252 {
                tunnel: w255 -> [w256 w263]
                tunnel: w254 -> [_ w262]
                tunnel: [w256 w261] -> w253
                tunnel: w251 -> [_ w260]
                tunnel: w250 -> [_ w259]
                tunnel: w249 -> [_ w258]
                frame False {
                }
                frame True {
                  n92 = Bundle By Name(cluster=w263, "Start Timestamp"=w262, "Operator"=w259, "Station ID"=w258, "Cartridge SN"=w260, "SW Version"="0.1.0") -> (w261:T6)
                }
              }
            }
            n93 = call "Update Cart Status.vi"("Selection"=status_update."Cartridge", "error in (no error)"=w203, "String"="TW in progress" ("Reagent"), "Array"=w191, "FP"=w192) -> ("error out"=w238:errorcluster)  [unwired: 6 in]
            n94 = call "Update Cart Status.vi"("Selection"=status_update."Main Status", "error in (no error)"=w238, "String"="Starting Thermal Wash" ("Reagent"), "FP"=w192) -> ("error out"=w234:errorcluster)  [unwired: 7 in]
            n95 = flat-sequence {
              tunnel: [w246] -> w190
              frame #0 {
                n96 = Tick Count (ms)() -> (millisecond timer value=w246:u32)
              }
            }
          }
          frame "SystemLeakTest" {
            # "unpress start button if failed"
            n97 = call "Update Cart Status.vi"("Selection"=status_update."Main Status", "String"="Checking Pressure and Leaks" ("Reagent"), "FP"=w268) -> ()  [unwired: 8 in, 1 out]
            n98 = call "Test Leak Rate.vi"("Main References"=w268, "error in (no error)"=w294, "Cart Array"=w273) -> ("error out"=w265:errorcluster, "Results"=w275:T8[], "RatePass"=w276:bool[], "VacPass"=w280:bool[])  [unwired: 5 in]
            n99 = call "Vacuum Level Test.vi"("FP"=w268, "Results"=w275, "VacPass"=w280, "Cart Array"=w273) -> ("Error String"=w278:string, "Pass/Fail Array"=w274:bool[])  [unwired: 6 in]
            n100 = And Array Elements(Boolean array=w274) -> (logical AND=w279:bool)
            n101 = case shown="False" w279 {
              selector: w279 -> [w310 _]
              tunnel: w278 -> [w312 _]
              tunnel: [w310 w317] -> w277
              tunnel: w276 -> [_ w324]
              tunnel: w268 -> [_ w323]
              tunnel: w275 -> [_ w322]
              tunnel: w273 -> [_ w316]
              frame False {
                n102 = Not(x=w310) -> (.not. x?=w314:bool)
                n103 = Concatenate Strings(w312, "Pressure Fail - make sure pump is on" ("string")) -> (w313:string)
                n104 = call "Display Message to User"("Enable"=w314, "Message"=w313) -> ()  [unwired: 8 in, 2 out]
              }
              frame True {
                n105 = call "Leak Test.vi"("FP"=w323, "Results"=w322, "RatePass"=w324, "Cart Array"=w316) -> ("Error String"=w321:string, "Pass/Fail Array"=w315:bool[])  [unwired: 6 in]
                n106 = And Array Elements(Boolean array=w315) -> (logical AND=w317:bool)
                n107 = Not(x=w317) -> (.not. x?=w320:bool)
                n108 = Concatenate Strings(w321, "\r\nPlease remove or fix cartrdige before restarting the test" ("string")) -> (w319:string)
                n109 = call "Display Message to User2"("Enable"=w320, "Message"=w319) -> ()  [unwired: 8 in, 2 out]
              }
            }
            n110 = Unbundle By Name(w268) -> ("Start TW"=w286:refnum<vi>)
            n111 = property class="Bool (strict)"(reference=w286, "Value"=w277) -> ()  [unwired: 1 in, 2 out]
            n112 = flat-sequence {
              tunnel: [w306] -> w267
              tunnel: w266 -> [w305]
              tunnel: w265 -> [w303]
              tunnel: [w300] -> w264
              frame #0 {
                n113 = Tick Count (ms)() -> (millisecond timer value=w300:u32)
                n114 = Subtract(x=w300, y=w305) -> (x-y=w297:u32)
                n115 = Divide(x=w297, y=u32 1000) -> (x/y=w299:dbl)
                n116 = call "Time Left Calc.vi"("Enum"=Time_elapsed."Update", "error in (no error)"=w303, "Time"=w299) -> ("error out"=w302:errorcluster)  [unwired: 6 in, 2 out]
                n117 = call "Time Left Calc.vi"("Enum"=Time_elapsed."Read", "error in (no error)"=w302) -> ("error out"=w308:errorcluster, "Time Left"=w307:u32)  [unwired: 7 in, 1 out]
                n118 = call "Time Left Calc.vi"("Enum"=Time_elapsed."Start", "error in (no error)"=w308, "Time"=w307) -> ("error out"=w306:errorcluster)  [unwired: 6 in, 2 out]
              }
            }
            n119 = for {
              N: 4 -> [_]
              tunnel: w283 -> [w327] mode=indexing
              tunnel: w273 -> [w328] mode=indexing
              tunnel: w275 -> [w326] mode=indexing
              tunnel: [w325] -> w281 mode=indexing
              n120 = case shown="True" w328 {
                tunnel: w327 -> [w329 w332]
                tunnel: w326 -> [_ w331]
                tunnel: [w329 w330] -> w325
                frame False {
                }
                frame True {
                  n121 = Bundle By Name(cluster=w332, "Pressure and Leak Test"=w331) -> (w330:T6)
                }
              }
            }
            n122 = Select(t=Process_State."Rinse Wells" ("State"), s=w289, f=Process_State."Prime System" ("State")) -> (s? t:f=w288:T5)
            n123 = Select(t=w288, s=w277, f=Process_State."Idle") -> (s? t:f=w271:T5)
            n124 = Select(t=w271, s=w272, f=Process_State."Idle") -> (s? t:f=w269:T5)
            n125 = Select(t=Process_State."Error", s=w267, f=w269) -> (s? t:f=w291:T5)
          }
          frame "Prime System" {
            n126 = call "Update Cart Status.vi"("Selection"=status_update."Main Status", "error in (no error)"=w337, "String"="Clearing wells and lines" ("Reagent"), "FP"=w342) -> ("error out"=w334:errorcluster)  [unwired: 7 in]
            n127 = call "Run Script.vi"("Script Name"="Drain All Wells" ("name or relative path"), "Main References"=w342, "error in (no error)"=w334) -> ("error out"=w346:errorcluster)  [unwired: 8 in]
            n128 = call "Update Cart Status.vi"("Selection"=status_update."Main Status", "error in (no error)"=w346, "String"="Priming input lines" ("Reagent"), "FP"=w342) -> ("error out"=w344:errorcluster)  [unwired: 7 in]
            n129 = call "Run Script.vi"("Script Name"="Prime Input Lines" ("name or relative path"), "Main References"=w342, "error in (no error)"=w344) -> ("error out"=w339:errorcluster)  [unwired: 8 in]
            n130 = for {
              tunnel: w348 -> [w373] mode=indexing
              tunnel: [w372] -> w347 mode=indexing
              n131 = Bundle By Name(cluster=w373, "Primed"=TRUE) -> (w372:T6)
            }
            n132 = flat-sequence {
              tunnel: w341 -> [w370]
              tunnel: [w363] -> w340
              tunnel: w339 -> [w362]
              tunnel: [w361] -> w338
              frame #0 {
                n133 = Tick Count (ms)() -> (millisecond timer value=w361:u32)
                n134 = Subtract(x=w361, y=w370) -> (x-y=w358:u32)
                n135 = Divide(x=w358, y=u32 1000) -> (x/y=w360:dbl)
                n136 = call "Time Left Calc.vi"("Enum"=Time_elapsed."Update", "error in (no error)"=w362, "Time"=w360) -> ("error out"=w369:errorcluster)  [unwired: 6 in, 2 out]
                n137 = call "Time Left Calc.vi"("Enum"=Time_elapsed."Read", "error in (no error)"=w369) -> ("error out"=w367:errorcluster, "Time Left"=w368:u32)  [unwired: 7 in, 1 out]
                n138 = call "Time Left Calc.vi"("Enum"=Time_elapsed."Start", "error in (no error)"=w367, "Time"=w368) -> ("error out"=w363:errorcluster)  [unwired: 6 in, 2 out]
              }
            }
            n139 = Select(t=Process_State."Rinse Wells" ("State"), s=w354, f=Process_State."Idle" ("State")) -> (s? t:f=w357:T5)
          }
          frame "Rinse Wells" {
            n140 = call "Update Cart Status.vi"("Selection"=status_update."Main Status", "error in (no error)"=w394, "String"="Draining Wells" ("Reagent"), "FP"=w378) -> ("error out"=w393:errorcluster)  [unwired: 7 in]
            n141 = call "Run Script.vi"("Script Name"="Drain All Wells" ("name or relative path"), "Main References"=w378, "error in (no error)"=w393) -> ("error out"=w379:errorcluster)  [unwired: 8 in]
            n142 = call "Update Cart Status.vi"("Selection"=status_update."Main Status", "error in (no error)"=w379, "String"="Rinsing Syringe" ("Reagent"), "FP"=w378) -> ("error out"=w386:errorcluster)  [unwired: 7 in]
            n143 = for {
              N: 3 -> [_]
              tunnel: "Rinse Syringe" ("name or relative path") -> [w420]
              shift-right: [w419] -> w383
              shift-left: w386 -> [w421]
              tunnel: w378 -> [w418]
              n144 = call "Run Script.vi"("Script Name"=w420, "Main References"=w418, "error in (no error)"=w421) -> ("error out"=w419:errorcluster)  [unwired: 8 in]
            }
            n145 = call "Update Cart Status.vi"("Selection"=status_update."Main Status", "error in (no error)"=w383, "String"="Rinsing all wells" ("Reagent"), "FP"=w378) -> ("error out"=w388:errorcluster)  [unwired: 7 in]
            n146 = for {
              N: 4 -> [_]
              shift-right: [w422] -> w375
              shift-left: w388 -> [w425]
              tunnel: w378 -> [w423]
              tunnel: "Rinse All Wells" ("Script Name") -> [w424]
              n147 = call "Run Script.vi"("Script Name"=w424, "Main References"=w423, "error in (no error)"=w425) -> ("error out"=w422:errorcluster)  [unwired: 8 in]
            }
            n148 = flat-sequence {
              tunnel: w377 -> [w417]
              tunnel: [w410] -> w376
              tunnel: w375 -> [w409]
              tunnel: [w408] -> w374
              frame #0 {
                n149 = Tick Count (ms)() -> (millisecond timer value=w408:u32)
                n150 = Subtract(x=w408, y=w417) -> (x-y=w405:u32)
                n151 = Divide(x=w405, y=u32 1000) -> (x/y=w407:dbl)
                n152 = call "Time Left Calc.vi"("Enum"=Time_elapsed."Update", "error in (no error)"=w409, "Time"=w407) -> ("error out"=w412:errorcluster)  [unwired: 6 in, 2 out]
                n153 = call "Time Left Calc.vi"("Enum"=Time_elapsed."Read", "error in (no error)"=w412) -> ("error out"=w415:errorcluster, "Time Left"=w414:u32)  [unwired: 7 in, 1 out]
                n154 = call "Time Left Calc.vi"("Enum"=Time_elapsed."Start", "error in (no error)"=w415, "Time"=w414) -> ("error out"=w410:errorcluster)  [unwired: 6 in, 2 out]
              }
            }
            n155 = Select(t=Process_State."PrePresTest" ("State"), s=w400, f=Process_State."Idle" ("State")) -> (s? t:f=w404:T5)
          }
          frame "Fill Wells" {
            # "Move to TW position if we are not doing liquid check"
            n156 = Index Array(array=w439, index=w443) -> (element=w442:T10)
            n157 = Unbundle By Name(w442) -> ("Reagent"=w433:string, "Bottle"=w441:T28)
            n158 = call "Update Cart Status.vi"("Selection"=status_update."Reagent", "error in (no error)"=w434, "String"=w433, "Array"=w432, "FP"=w430) -> ("error out"=w431:errorcluster)  [unwired: 6 in]
            n159 = case shown="\"Bottle 1\"" w441 {
              tunnel: [Bottles."Bottle 1" ("Bottle X") Bottles."Bottle 2" ("Bottle X") Bottles."Bottle 3" ("Bottle X") Bottles."H2O" ("Bottle X")] -> w436
              frame "Bottle 1" {
              }
              frame "Bottle 2" {
              }
              frame "Bottle 3" {
              }
              frame "Bottle 4" {
              }
            }
            n160 = for {
              N: 4 -> [_]
              tunnel: w432 -> [w478] mode=indexing
              tunnel: w436 -> [w479]
              shift-right: [w480] -> w440
              shift-left: w431 -> [w476]
              tunnel: w430 -> [w475]
              tunnel: w433 -> [w474]
              i -> [w477]
              n161 = case shown="True" w478 {
                tunnel: w476 -> [w481 w490]
                tunnel: w477 -> [_ w482]
                tunnel: [w481 w493] -> w480
                tunnel: w479 -> [_ w491]
                tunnel: w475 -> [_ w487]
                tunnel: w474 -> [_ w485]
                frame False {
                }
                frame True {
                  n162 = Increment(x=w482) -> (x+1=w484:i32)
                  n163 = Format Into String(format string="Filling well %d with %s", w484, w485) -> (resulting string=w483:string)  [unwired: 2 in, 1 out]
                  n164 = call "Update Cart Status.vi"("Selection"=status_update."Main Status", "error in (no error)"=w490, "String"=w483, "FP"=w487) -> ("error out"=w489:errorcluster)  [unwired: 7 in]
                  n165 = call "Run Script.vi"("Script Name"="Fill Well_X Reagent_X" ("name or relative path"), "Main References"=w487, "error in (no error)"=w489, "Drain X"=w482, "Well X"=w482, "Bottle X"=w491) -> ("error out"=w493:errorcluster)  [unwired: 5 in]
                }
              }
            }
            n166 = case shown="True" FALSE {
              tunnel: w440 -> [w465 w468]
              tunnel: [w465 w467] -> w427
              tunnel: w430 -> [_ w466]
              frame False {
              }
              frame True {
                n167 = call "Run Script.vi"("Script Name"="Move to TW" ("name or relative path"), "Main References"=w466, "error in (no error)"=w468) -> ("error out"=w467:errorcluster)  [unwired: 8 in]
              }
            }
            n168 = flat-sequence {
              tunnel: [w458] -> w429
              tunnel: [w457] -> w428
              tunnel: w427 -> [w453]
              tunnel: w426 -> [w452]
              frame #0 {
                n169 = Tick Count (ms)() -> (millisecond timer value=w457:u32)
                n170 = Subtract(x=w457, y=w452) -> (x-y=w454:u32)
                n171 = Divide(x=w454, y=u32 1000) -> (x/y=w456:dbl)
                n172 = call "Time Left Calc.vi"("Enum"=Time_elapsed."Update", "error in (no error)"=w453, "Time"=w456) -> ("error out"=w460:errorcluster)  [unwired: 6 in, 2 out]
                n173 = call "Time Left Calc.vi"("Enum"=Time_elapsed."Read", "error in (no error)"=w460) -> ("error out"=w463:errorcluster, "Time Left"=w462:u32)  [unwired: 7 in, 1 out]
                n174 = call "Time Left Calc.vi"("Enum"=Time_elapsed."Start", "error in (no error)"=w463, "Time"=w462) -> ("error out"=w458:errorcluster)  [unwired: 6 in, 2 out]
              }
            }
            n175 = Select(t=Process_State."Apply Pressure" ("State"), s=w447, f=Process_State."Idle" ("State")) -> (s? t:f=w445:T5)
            n176 = Select(t=Process_State."Error" ("State"), s=w427, f=w445) -> (s? t:f=w444:T5)
          }
          frame "PrePresTest" {
            n177 = Unbundle By Name(w506) -> ("Config"=w513:refnum<vi>)
            n178 = property class="Clust (strict)"(reference=w513) -> ("Value"=w512:T1)  [unwired: 1 in, 2 out]
            n179 = Unbundle By Name(w512) -> ("TW Position"=w507:dbl, "Load Position"=w499:dbl)
            n180 = call "Update Cart Status.vi"("Selection"=status_update."Main Status", "error in (no error)"=w515, "String"="Testing for leaks and clogs", "FP"=w506) -> ("error out"=w508:errorcluster)  [unwired: 7 in]
            n181 = call "Detect Transition to TW.vi"("Main References"=w506, "error in (no error)"=w508, "Cart Array"=w502) -> ("error out"=w497:errorcluster, "Analysis"=w500:T7[])  [unwired: 7 in]
            n182 = case shown="True" TRUE {
              tunnel: w500 -> [_ w550]
              tunnel: w500 -> [_ w549]
              tunnel: w502 -> [w545 w548]
              tunnel: w506 -> [_ w547]
              tunnel: [w545 w546] -> w505
              frame False {
              }
              frame True {
                n183 = for {
                  tunnel: w550 -> [w556] mode=indexing
                  tunnel: w549 -> [w554] mode=indexing
                  tunnel: w548 -> [w555] mode=indexing
                  tunnel: w547 -> [w553]
                  tunnel: [w551] -> w546 mode=indexing
                  i -> [w552]
                  n184 = case shown="True" w555 {
                    selector: w555 -> [w557 _]
                    tunnel: w556 -> [_ w573]
                    tunnel: w554 -> [_ w572]
                    tunnel: w553 -> [_ w569]
                    tunnel: w552 -> [_ w568]
                    tunnel: [w557 w566] -> w551
                    frame False {
                    }
                    frame True {
                      n185 = Unbundle By Name(w573) -> ("Pressure"=w571:bool)
                      n186 = Unbundle By Name(w572) -> ("Decay"=w559:bool, "Pressure"=w570:bool)
                      n187 = Increment(x=w568) -> (x+1=w565:i32)
                      n188 = And(x=w571, y=w570) -> (x .and. y?=w560:bool)
                      n189 = Select(t="Test Passed" ("String"), s=w559, f="Clog Detected" ("String")) -> (s? t:f=w562:string)
                      n190 = And(x=w560, y=w559) -> (x .and. y?=w558:bool)
                      n191 = Select(t=w562, s=w560, f="Pressure Level Fail" ("String")) -> (s? t:f=w567:string)
                      n192 = case shown="False" w558 {
                        selector: w558 -> [w575 w579]
                        tunnel: w569 -> [w578 _]
                        tunnel: w565 -> [w577 _]
                        tunnel: w567 -> [w576 _]
                        tunnel: [w575 w579] -> w566
                        frame False {
                          n193 = call "Update 1 Cart Status.vi"("Selection"=Update_Single_Cart."Cart Status", "FP"=w578, "String"=w576, "Cartridge"=w577) -> ()  [unwired: 7 in, 1 out]
                        }
                        frame True {
                        }
                      }
                    }
                  }
                }
              }
            }
            n194 = flat-sequence {
              tunnel: [w530] -> w496
              tunnel: [w529] -> w495
              tunnel: w497 -> [w525]
              tunnel: w494 -> [w524]
              frame #0 {
                n195 = Tick Count (ms)() -> (millisecond timer value=w529:u32)
                n196 = Subtract(x=w529, y=w524) -> (x-y=w526:u32)
                n197 = Divide(x=w526, y=u32 1000) -> (x/y=w528:dbl)
                n198 = call "Time Left Calc.vi"("Enum"=Time_elapsed."Update", "error in (no error)"=w525, "Time"=w528) -> ("error out"=w532:errorcluster)  [unwired: 6 in, 2 out]
                n199 = call "Time Left Calc.vi"("Enum"=Time_elapsed."Read", "error in (no error)"=w532) -> ("error out"=w535:errorcluster, "Time Left"=w534:u32)  [unwired: 7 in, 1 out]
                n200 = call "Time Left Calc.vi"("Enum"=Time_elapsed."Start", "error in (no error)"=w535, "Time"=w534) -> ("error out"=w530:errorcluster)  [unwired: 6 in, 2 out]
              }
            }
            n201 = case shown="False" w503 {
              tunnel: w507 -> [w539 _]
              tunnel: w496 -> [w538 w543]
              tunnel: [w537 w542] -> w498
              tunnel: w499 -> [_ w541]
              frame True {
                n202 = call "Zaber Manager.vi"("Action"=Mot_Stage_Mngr."Abs Move", "Value"=w539, "error in (no error)"=w538) -> ("error out"=w537:errorcluster)  [unwired: 6 in, 6 out]
              }
              frame False {
                n203 = call "Zaber Manager.vi"("Action"=Mot_Stage_Mngr."Abs Move", "Value"=w541, "error in (no error)"=w543) -> ("error out"=w542:errorcluster)  [unwired: 6 in, 6 out]
              }
            }
            n204 = for {
              N: 4 -> [_]
              tunnel: w510 -> [w584] mode=indexing
              tunnel: [w585] -> w509 mode=indexing
              tunnel: w511 -> [w580]
              tunnel: w500 -> [w581] mode=indexing
              n205 = Unbundle By Name(w584) -> ("Test Array Pre"=w583:T7[])
              n206 = Insert Into Array(array=w583, index=w580, new element=w581) -> (w582:T7[])
              n207 = Bundle By Name(cluster=w584, "Test Array Pre"=w582) -> (w585:T6)
            }
            n208 = Select(t=Process_State."Fill Wells" ("State"), s=w503, f=Process_State."Idle" ("State")) -> (s? t:f=w519:T5)
            n209 = Select(t=Process_State."Error" ("State"), s=w498, f=w519) -> (s? t:f=w518:T5)
          }
          frame "Apply Pressure" {
            n210 = call "Update Cart Status.vi"("Selection"=status_update."Main Status", "error in (no error)"=w599, "String"="Applying pressure" ("Reagent"), "FP"=w594) -> ("error out"=w598:errorcluster)  [unwired: 7 in]
            n211 = Index Array(array=w605, index=w611) -> (element=w612:T10)
            n212 = Unbundle By Name(w612) -> ("Wash Time(s)"=w606:dbl)
            n213 = call "Denkovi Manager.vi"("Action"=Denkovi_Mngr."Pres ON", "error in (no error)"=w598, "Relays In"=w593) -> ("error out"=w610:errorcluster)  [unwired: 6 in, 2 out]
            n214 = flat-sequence {
              tunnel: w610 -> [w622]
              tunnel: [w622] -> w609
              tunnel: [w621] -> w608
              frame #0 {
                n215 = Tick Count (ms)() -> (millisecond timer value=w621:u32)
              }
            }
            n216 = while {
              tunnel: w609 -> [w638]
              tunnel: [w632] -> w604
              tunnel: w608 -> [w644]
              tunnel: w607 -> [_]
              tunnel: w606 -> [w643]
              tunnel: w594 -> [w631]
              tunnel: w593 -> [w630]
              tunnel: [w623] -> w586
              stop <- w640 stop-if-true
              n217 = call "DAQ Manager.vi"("DAQ Mngr Action"=DAQ_Mngr."Analyze Pressure", "error in (no error)"=w638) -> ("error out"=w637:errorcluster)  [unwired: 7 in, 6 out]
              n218 = flat-sequence {
                tunnel: w637 -> [w646]
                tunnel: [w646] -> w633
                tunnel: [w645] -> w623
                frame #0 {
                  n219 = Tick Count (ms)() -> (millisecond timer value=w645:u32)
                }
              }
              n220 = expression code="x*1000"(w643) -> (w629:dbl)
              n221 = Subtract(x=w623, y=w644) -> (x-y=w625:u32)
              n222 = Subtract(x=w629, y=w625) -> (x-y=w628:dbl)
              n223 = expression code="x/1000"(w625) -> (w624:u32)
              n224 = expression code="x/1000"(w628) -> (w627:dbl)
              n225 = global read "Main Globals.vi" "Cancel"() -> (w642:bool)
              n226 = call "Time Left Calc.vi"("Enum"=Time_elapsed."Update", "Time"=w624) -> ()  [unwired: 7 in, 3 out]
              n227 = Format Into String(format string="%.1f seconds", w627) -> (resulting string=w634:string)  [unwired: 2 in, 1 out]
              n228 = Greater?(x=w625, y=w629) -> (0:w641:bool)
              n229 = Compound Arithmetic op=OR(w641, w642) -> (w640:bool)
              n230 = call "Update Cart Status.vi"("Selection"=status_update."Cartridge", "error in (no error)"=w633, "String"=w634, "Array"=w630, "FP"=w631) -> ("error out"=w632:errorcluster)  [unwired: 6 in]
            }
            n231 = call "Denkovi Manager.vi"("Action"=Denkovi_Mngr."Vent&Close", "error in (no error)"=w604, "Relays In"=w593) -> ("error out"=w596:errorcluster)  [unwired: 6 in, 2 out]
            n232 = call "Update Cart Status.vi"("Selection"=status_update."Cartridge", "error in (no error)"=w596, "String"="TW in progress", "Array"=w593, "FP"=w594) -> ("error out"=w592:errorcluster)  [unwired: 6 in]
            n233 = call "Time Left Calc.vi"("Enum"=Time_elapsed."Read", "error in (no error)"=w592) -> ("error out"=w590:errorcluster, "Time Left"=w588:u32)  [unwired: 7 in, 1 out]
            n234 = call "Time Left Calc.vi"("Enum"=Time_elapsed."Start", "error in (no error)"=w590, "Time"=w588) -> ("error out"=w587:errorcluster)  [unwired: 6 in, 2 out]
            n235 = Select(t=Process_State."Drain&Rinse" ("State"), s=w617, f=Process_State."Idle" ("State")) -> (s? t:f=w615:T5)
            n236 = Select(t=Process_State."Error" ("State"), s=w587, f=w615) -> (s? t:f=w614:T5)
          }
          frame "PostPresTest" {
            n237 = Unbundle By Name(w661) -> ("Config"=w667:refnum<vi>)
            n238 = property class="Clust (strict)"(reference=w667) -> ("Value"=w666:T1)  [unwired: 1 in, 2 out]
            n239 = Unbundle By Name(w666) -> ("Load Position"=w662:dbl)
            n240 = call "Update Cart Status.vi"("Selection"=status_update."Main Status", "error in (no error)"=w669, "String"="Testing for leaks and clogs", "FP"=w661) -> ("error out"=w655:errorcluster)  [unwired: 7 in]
            n241 = call "Detect Transition to Load.vi"("Main References"=w661, "error in (no error)"=w655, "Cart Array"=w647) -> ("error out"=w653:errorcluster, "Analysis"=w654:T7[])  [unwired: 7 in]
            n242 = case shown="True" FALSE {
              tunnel: w654 -> [_ w701]
              tunnel: w654 -> [_ w700]
              tunnel: w647 -> [w696 w699]
              tunnel: w661 -> [_ w698]
              tunnel: [w696 w697] -> w660
              frame False {
              }
              frame True {
                n243 = for {
                  tunnel: w701 -> [w707] mode=indexing
                  tunnel: w700 -> [w705] mode=indexing
                  tunnel: w699 -> [w706] mode=indexing
                  tunnel: w698 -> [w704]
                  tunnel: [w702] -> w697 mode=indexing
                  i -> [w703]
                  n244 = case shown="True" w706 {
                    selector: w706 -> [w708 _]
                    tunnel: w707 -> [_ w726]
                    tunnel: w705 -> [_ w725]
                    tunnel: w704 -> [_ w720]
                    tunnel: w703 -> [_ w718]
                    tunnel: [w708 w714] -> w702
                    frame False {
                    }
                    frame True {
                      n245 = Unbundle By Name(w726) -> ("Transition"=w724:bool, "Pressure"=w722:bool)
                      n246 = Unbundle By Name(w725) -> ("Transition"=w723:bool, "Pressure"=w721:bool)
                      n247 = Increment(x=w718) -> (x+1=w713:i32)
                      n248 = And(x=w722, y=w721) -> (x .and. y?=w717:bool)
                      n249 = And(x=w724, y=w723) -> (x .and. y?=w716:bool)
                      n250 = Select(t="Test Passed" ("String"), s=w716, f="Clog Detected" ("String")) -> (s? t:f=w710:string)
                      n251 = And(x=w716, y=w717) -> (x .and. y?=w719:bool)
                      n252 = Select(t=w710, s=w717, f="Pressure Level Fail" ("String")) -> (s? t:f=w715:string)
                      n253 = case shown="False" w719 {
                        selector: w719 -> [w728 w732]
                        tunnel: w720 -> [w731 _]
                        tunnel: w713 -> [w730 _]
                        tunnel: w715 -> [w729 _]
                        tunnel: [w728 w732] -> w714
                        frame False {
                          n254 = call "Update 1 Cart Status.vi"("Selection"=Update_Single_Cart."Cart Status", "FP"=w731, "String"=w729, "Cartridge"=w730) -> ()  [unwired: 7 in, 1 out]
                        }
                        frame True {
                        }
                      }
                    }
                  }
                }
              }
            }
            n255 = call "Denkovi Manager.vi"("Action"=Denkovi_Mngr."Vent&Close", "error in (no error)"=w653, "Relays In"=w647) -> ("error out"=w651:errorcluster)  [unwired: 6 in, 2 out]
            n256 = flat-sequence {
              tunnel: [w684] -> w650
              tunnel: [w683] -> w649
              tunnel: w651 -> [w679]
              tunnel: w648 -> [w678]
              frame #0 {
                n257 = Tick Count (ms)() -> (millisecond timer value=w683:u32)
                n258 = Subtract(x=w683, y=w678) -> (x-y=w680:u32)
                n259 = Divide(x=w680, y=u32 1000) -> (x/y=w682:dbl)
                n260 = call "Time Left Calc.vi"("Enum"=Time_elapsed."Update", "error in (no error)"=w679, "Time"=w682) -> ("error out"=w686:errorcluster)  [unwired: 6 in, 2 out]
                n261 = call "Time Left Calc.vi"("Enum"=Time_elapsed."Read", "error in (no error)"=w686) -> ("error out"=w689:errorcluster, "Time Left"=w688:u32)  [unwired: 7 in, 1 out]
                n262 = call "Time Left Calc.vi"("Enum"=Time_elapsed."Start", "error in (no error)"=w689, "Time"=w688) -> ("error out"=w684:errorcluster)  [unwired: 6 in, 2 out]
              }
            }
            n263 = for {
              N: 4 -> [_]
              tunnel: w664 -> [w737] mode=indexing
              tunnel: [w738] -> w663 mode=indexing
              tunnel: w665 -> [w733]
              tunnel: w654 -> [w734] mode=indexing
              n264 = Unbundle By Name(w737) -> ("Test Array Post"=w736:T7[])
              n265 = Insert Into Array(array=w736, index=w733, new element=w734) -> (w735:T7[])
              n266 = Bundle By Name(cluster=w737, "Test Array Post"=w735) -> (w738:T6)
            }
            n267 = case shown="True" w656 {
              tunnel: w662 -> [_ w694]
              tunnel: w650 -> [w691 w693]
              tunnel: [w691 w692] -> w658
              frame False {
              }
              frame True {
                n268 = call "Zaber Manager.vi"("Action"=Mot_Stage_Mngr."Abs Move", "Value"=w694, "error in (no error)"=w693) -> ("error out"=w692:errorcluster)  [unwired: 6 in, 6 out]
              }
            }
            n269 = Select(t=Process_State."Drain&Rinse" ("State"), s=w656, f=Process_State."Idle" ("State")) -> (s? t:f=w673:T5)
            n270 = Select(t=Process_State."Error" ("State"), s=w658, f=w673) -> (s? t:f=w672:T5)
          }
          frame "Drain&Rinse" {
            n271 = call "Update Cart Status.vi"("Selection"=status_update."Main Status", "error in (no error)"=w749, "String"="Draining Wells", "FP"=w750) -> ("error out"=w748:errorcluster)  [unwired: 7 in]
            n272 = Unbundle By Name(w750) -> ("Config"=w760:refnum<vi>)
            n273 = property class="Clust (strict)"(reference=w760) -> ("Value"=w759:T1)  [unwired: 1 in, 2 out]
            n274 = Unbundle By Name(w759) -> ("Load Position"=w758:dbl)
            n275 = Index Array(array=w767, index=w769) -> (element=w775:T10)
            n276 = call "Zaber Manager.vi"("Action"=Mot_Stage_Mngr."Abs Move", "Value"=w758, "error in (no error)"=w748) -> ("error out"=w754:errorcluster)  [unwired: 6 in, 6 out]
            n277 = Unbundle By Name(w775) -> ("# of Rinses"=w744:i16)
            n278 = for {
              N: 4 -> [_]
              shift-right: [w796] -> w753
              shift-left: w754 -> [w797]
              tunnel: w755 -> [w795] mode=indexing
              tunnel: w750 -> [w793]
              tunnel: "Drain Well X" ("Script Name") -> [w792]
              i -> [w794]
              n279 = case shown="True" w795 {
                tunnel: w797 -> [w798 w803]
                tunnel: [w798 w801] -> w796
                tunnel: w794 -> [_ w802]
                tunnel: w793 -> [_ w800]
                tunnel: w792 -> [_ w799]
                frame False {
                }
                frame True {
                  n280 = call "Run Script.vi"("Script Name"=w799, "Main References"=w800, "error in (no error)"=w803, "Drain X"=w802, "Well X"=w802) -> ("error out"=w801:errorcluster)  [unwired: 6 in]
                }
              }
            }
            n281 = case shown="False" w745 {
              tunnel: w744 -> [_ w791]
              tunnel: [i16 1 ("# of Rinses") w791] -> w743
              frame False {
              }
              frame True {
              }
            }
            n282 = case shown="Default" w743 {
              selector: w743 -> [_ w808]
              tunnel: w755 -> [_ w811]
              tunnel: w753 -> [w804 w805]
              tunnel: w750 -> [_ w810]
              tunnel: [w804 w809] -> w742
              tunnel: "Rinse Well X step1" ("Script Name") -> [_ w807]
              tunnel: "Rinse Well X step3" ("Script Name") -> [_ w806]
              frame 0 {
                # "skip rinsing if # of rinses is 0"
              }
              frame Default {
                n283 = for {
                  N: w808 -> [w820]
                  tunnel: w811 -> [w812]
                  tunnel: w810 -> [w813]
                  shift-right: [w822] -> w809
                  shift-left: w805 -> [w825]
                  tunnel: w807 -> [w816]
                  tunnel: w806 -> [w815]
                  i -> [w818]
                  n284 = Increment(x=w818) -> (x+1=w817:i32)
                  n285 = Format Into String(format string="Rinsing wells %d/%d", w817, w820) -> (resulting string=w819:string)  [unwired: 2 in, 1 out]
                  n286 = call "Update Cart Status.vi"("Selection"=status_update."Main Status", "error in (no error)"=w825, "String"=w819, "FP"=w813) -> ("error out"=w824:errorcluster)  [unwired: 7 in]
                  n287 = for {
                    N: 4 -> [_]
                    shift-right: [w844] -> w814
                    shift-left: w824 -> [w845]
                    tunnel: w812 -> [w843] mode=indexing
                    tunnel: w813 -> [w841]
                    tunnel: w816 -> [w840]
                    i -> [w842]
                    n288 = case shown="True" w843 {
                      tunnel: w845 -> [w846 w851]
                      tunnel: [w846 w849] -> w844
                      tunnel: w842 -> [_ w850]
                      tunnel: w841 -> [_ w848]
                      tunnel: w840 -> [_ w847]
                      frame False {
                      }
                      frame True {
                        n289 = call "Run Script.vi"("Script Name"=w847, "Main References"=w848, "error in (no error)"=w851, "Drain X"=w850, "Well X"=w850) -> ("error out"=w849:errorcluster)  [unwired: 6 in]
                      }
                    }
                  }
                  n290 = for {
                    N: 4 -> [_]
                    shift-right: [w832] -> w822
                    shift-left: w814 -> [w833]
                    tunnel: w812 -> [w831] mode=indexing
                    tunnel: w813 -> [w829]
                    tunnel: w815 -> [w828]
                    i -> [w830]
                    n291 = case shown="True" w831 {
                      tunnel: w833 -> [w834 w839]
                      tunnel: [w834 w837] -> w832
                      tunnel: w830 -> [_ w838]
                      tunnel: w829 -> [_ w836]
                      tunnel: w828 -> [_ w835]
                      frame False {
                      }
                      frame True {
                        n292 = call "Run Script.vi"("Script Name"=w835, "Main References"=w836, "error in (no error)"=w839, "Drain X"=w838, "Well X"=w838) -> ("error out"=w837:errorcluster)  [unwired: 6 in]
                      }
                    }
                  }
                }
              }
            }
            n293 = Increment(x=w769) -> (x+1=w768:i32)
            n294 = Array Size(array=w767) -> (size(s)=w770:i32)
            n295 = Greater?(x=w770, y=w768) -> (0:w766:bool)
            n296 = flat-sequence {
              tunnel: [w783] -> w741
              tunnel: [w782] -> w740
              tunnel: w742 -> [w778]
              tunnel: w739 -> [w777]
              frame #0 {
                n297 = Tick Count (ms)() -> (millisecond timer value=w782:u32)
                n298 = Subtract(x=w782, y=w777) -> (x-y=w779:u32)
                n299 = Divide(x=w779, y=u32 1000) -> (x/y=w781:dbl)
                n300 = call "Time Left Calc.vi"("Enum"=Time_elapsed."Update", "error in (no error)"=w778, "Time"=w781) -> ("error out"=w785:errorcluster)  [unwired: 6 in, 2 out]
                n301 = call "Time Left Calc.vi"("Enum"=Time_elapsed."Read", "error in (no error)"=w785) -> ("error out"=w788:errorcluster, "Time Left"=w787:u32)  [unwired: 7 in, 1 out]
                n302 = call "Time Left Calc.vi"("Enum"=Time_elapsed."Start", "error in (no error)"=w788, "Time"=w787) -> ("error out"=w783:errorcluster)  [unwired: 6 in, 2 out]
              }
            }
            n303 = Select(t=Process_State."Fill Wells" ("State"), s=w766, f=Process_State."Dry" ("State")) -> (s? t:f=w764:T5)
            n304 = Select(t=w764, s=w745, f=Process_State."Idle") -> (s? t:f=w762:T5)
            n305 = Select(t=Process_State."Error" ("State"), s=w741, f=w762) -> (s? t:f=w771:T5)
          }
          frame "Dry" {
            n306 = Unbundle By Name(w858) -> ("Config"=w864:refnum<vi>)
            n307 = property class="Clust (strict)"(reference=w864) -> ("Value"=w862:T1)  [unwired: 1 in, 2 out]
            n308 = Unbundle By Name(w862) -> ("Dry Time(s)"=w861:dbl, "Load Position"=w863:dbl)
            n309 = Format Into String(format string="Drying capillaries for %ds", w861) -> (resulting string=w859:string)  [unwired: 2 in, 1 out]
            n310 = call "Update Cart Status.vi"("Selection"=status_update."Main Status", "error in (no error)"=w866, "String"=w859, "FP"=w858) -> ("error out"=w865:errorcluster)  [unwired: 7 in]
            n311 = call "Zaber Manager.vi"("Action"=Mot_Stage_Mngr."Abs Move", "Value"=w863, "error in (no error)"=w865) -> ("error out"=w872:errorcluster)  [unwired: 6 in, 6 out]
            n312 = call "Denkovi Manager.vi"("Action"=Denkovi_Mngr."Pres ON", "error in (no error)"=w872, "Relays In"=w857) -> ("error out"=w884:errorcluster)  [unwired: 6 in, 2 out]
            n313 = flat-sequence {
              tunnel: w884 -> [w888]
              tunnel: [w888] -> w883
              tunnel: [w887] -> w882
              frame #0 {
                n314 = Tick Count (ms)() -> (millisecond timer value=w887:u32)
              }
            }
            n315 = while {
              tunnel: w883 -> [w905]
              tunnel: [w901] -> w880
              tunnel: w882 -> [w910]
              tunnel: w857 -> [w898]
              tunnel: w881 -> [_]
              tunnel: w861 -> [w909]
              tunnel: w858 -> [w899]
              tunnel: [w889] -> w852
              stop <- w906 stop-if-true
              n316 = call "DAQ Manager.vi"("DAQ Mngr Action"=DAQ_Mngr."Analyze Pressure", "error in (no error)"=w905) -> ("error out"=w904:errorcluster)  [unwired: 7 in, 6 out]
              n317 = flat-sequence {
                tunnel: w904 -> [w912]
                tunnel: [w912] -> w902
                tunnel: [w911] -> w889
                frame #0 {
                  n318 = Tick Count (ms)() -> (millisecond timer value=w911:u32)
                }
              }
              n319 = expression code="x*1000"(w909) -> (w893:dbl)
              n320 = Subtract(x=w889, y=w910) -> (x-y=w892:u32)
              n321 = Subtract(x=w893, y=w892) -> (x-y=w897:dbl)
              n322 = expression code="x/1000"(w892) -> (w891:u32)
              n323 = expression code="x/1000"(w897) -> (w896:dbl)
              n324 = Greater?(x=w892, y=w893) -> (0:w907:bool)
              n325 = call "Time Left Calc.vi"("Enum"=Time_elapsed."Update", "Time"=w891) -> ()  [unwired: 7 in, 3 out]
              n326 = Format Into String(format string="%.1f seconds", w896) -> (resulting string=w894:string)  [unwired: 2 in, 1 out]
              n327 = global read "Main Globals.vi" "Cancel"() -> (w908:bool)
              n328 = call "Update Cart Status.vi"("Selection"=status_update."Cartridge", "error in (no error)"=w902, "String"=w894, "Array"=w898, "FP"=w899) -> ("error out"=w901:errorcluster)  [unwired: 6 in]
              n329 = Compound Arithmetic op=OR(w907, w908) -> (w906:bool)
            }
            n330 = call "Denkovi Manager.vi"("Action"=Denkovi_Mngr."Vent&Close", "error in (no error)"=w880, "Relays In"=w857) -> ("error out"=w853:errorcluster)  [unwired: 6 in, 2 out]
            n331 = Select(t=Process_State."Report" ("State"), s=w869, f=Process_State."Idle" ("State")) -> (s? t:f=w875:T5)
            n332 = call "Time Left Calc.vi"("Enum"=Time_elapsed."Start", "error in (no error)"=w853, "Time"=u32 0) -> ("error out"=w854:errorcluster)  [unwired: 6 in, 2 out]
            n333 = Select(t=Process_State."Error" ("State"), s=w854, f=w875) -> (s? t:f=w874:T5)
          }
          frame "Error" {
            # "TODO:  handle errors\nask user to remove cartridges"
            n334 = call "Data Logger.vi"("Action"=enum16{"Init", "Save", "Close"}."Close", "error in"=w915) -> ("error out"=w914:errorcluster)  [unwired: 9 in]
            n335 = Unbundle By Name(w918) -> ("Cartridges"=w923:refnum<vi>)
            n336 = Unbundle By Name(w918) -> ("Start TW"=w925:refnum<vi>)
            n337 = property class="Bool (strict)"(reference=w925, "Value"=FALSE) -> ()  [unwired: 1 in, 2 out]
            n338 = property class="Clust (strict)"(reference=w923) -> (reference out=w920:refnum<vi>, "Value"=w922:T26)  [unwired: 1 in, 1 out]
            n339 = Bundle By Name(cluster=w922, "Current Status"="Error has occured.  Process aborted") -> (w919:T26)
            n340 = property class="Clust (strict)"(reference=w920, "Value"=w919) -> ()  [unwired: 1 in, 2 out]
          }
          frame "Abort" {
            n341 = call "Update Cart Status.vi"("Selection"=status_update."Main Status", "error in (no error)"=w950, "String"="Aborting Run" ("Reagent"), "FP"=w938) -> ("error out"=w939:errorcluster)  [unwired: 7 in]
            n342 = call "Zaber Manager.vi"("Action"=Mot_Stage_Mngr."Home", "error in (no error)"=w939) -> ("error out"=w946:errorcluster)  [unwired: 7 in, 6 out]
            n343 = call "Denkovi Manager.vi"("Action"=Denkovi_Mngr."Set Peristaltic", "error in (no error)"=w946, "Relays In"=bool[] [FALSE, FALSE, FALSE, FALSE, FALSE, FALSE, FALSE, FALSE, FALSE, FALSE, FALSE, FALSE, FALSE, FALSE, FALSE, FALSE]) -> ("error out"=w945:errorcluster)  [unwired: 6 in, 2 out]
            n344 = call "Denkovi Manager.vi"("Action"=Denkovi_Mngr."Vent&Close", "error in (no error)"=w945, "Relays In"=bool[] [TRUE, TRUE, TRUE, TRUE, FALSE, FALSE, FALSE, FALSE, FALSE, FALSE, FALSE, FALSE, FALSE, FALSE, FALSE, FALSE]) -> ("error out"=w944:errorcluster)  [unwired: 6 in, 2 out]
            n345 = call "Tecan Mngr.vi"("Mngr Action"=Tricon_Mngr."Start Pump", "Pump Data"=T22 {"Syringe Pos"=0, "Rate"=60.0, "Volume"=0.0, "Valve"=enum."Waste", "Action"=enum."Withdraw", "Move Type"=enum."Abs", "Init"=TRUE, "Empty Syr."=FALSE, "Full Fill"=FALSE, "Units"=enum."ul/s"}, "Pump Config"=w937, "error in (no error)"=w944) -> ("error out"=w934:errorcluster)  [unwired: 6 in, 5 out]
            n346 = call "DAQ Manager.vi"("DAQ Mngr Action"=DAQ_Mngr."Pinch Valve Disengage", "error in (no error)"=w934) -> ("error out"=w933:errorcluster)  [unwired: 7 in, 6 out]
            n347 = call "Data Logger.vi"("Action"=enum16{"Init", "Save", "Close"}."Close", "error in"=w933) -> ("error out"=w941:errorcluster)  [unwired: 9 in]
          }
          frame "Report" {
            n348 = Get Date/Time String(date format (0)=enum16{"short", "long", "abbreviated"}."short") -> (date string=w974:string, time string=w973:string)  [unwired: 2 in]
            n349 = Concatenate Strings(w974, "   " ("string"), w973) -> (w971:string)
            n350 = for {
              tunnel: w970 -> [w1006] mode=indexing
              tunnel: w971 -> [w1005]
              tunnel: [w1004] -> w968 mode=indexing
              tunnel: w962 -> [w1003] mode=indexing
              n351 = case shown="True" w1003 {
                tunnel: w1006 -> [w1007 w1010]
                tunnel: w1005 -> [_ w1009]
                tunnel: [w1007 w1008] -> w1004
                frame False {
                }
                frame True {
                  n352 = Bundle By Name(cluster=w1010, "Finish Timestamp"=w1009) -> (w1008:T6)
                }
              }
            }
            n353 = call "Data Logger.vi"("Action"=enum16{"Init", "Save", "Close"}."Close", "error in"=w966) -> ("error out"=w965:errorcluster)  [unwired: 9 in]
            n354 = for {
              N: 4 -> [_]
              tunnel: w965 -> [w986]
              tunnel: [w985] -> w969
              tunnel: w962 -> [w984] mode=indexing
              tunnel: w968 -> [w983] mode=indexing
              tunnel: w964 -> [w982]
              i -> [w981]
              n355 = case shown="True" w984 {
                tunnel: w986 -> [w987 w1002]
                tunnel: [w987 w999] -> w985
                tunnel: w983 -> [_ w1001]
                tunnel: w982 -> [_ w998]
                tunnel: w981 -> [_ w996]
                frame False {
                }
                frame True {
                  n356 = call "Create Summary File.vi"("FP"=w998, "error in"=w1002, "Report"=w1001) -> ("error out"=w1000:errorcluster, "Vac?"=w990:bool, "Pass/Fail"=w995:bool)  [unwired: 5 in, 1 out]
                  n357 = Increment(x=w996) -> (x+1=w992:i32)
                  n358 = Select(t="Pass" ("String"), s=w995, f="Clog" ("String")) -> (s? t:f=w991:string)
                  n359 = Select(t=w991, s=w990, f="Pressure Fail") -> (s? t:f=w988:string)
                  n360 = call "Update 1 Cart Status.vi"("Selection"=Update_Single_Cart."Cart Reagent", "FP"=w998, "error in (no error)"=w1000, "String"=w988, "Cartridge"=w992) -> ("error out"=w999:errorcluster)  [unwired: 6 in]
                }
              }
            }
          }
          frame "Finish" {
            n361 = Unbundle By Name(w1015) -> ("Config"=w1021:refnum<vi>)
            n362 = Unbundle By Name(w1015) -> ("Start TW"=w1030:refnum<vi>)
            n363 = property class="Clust (strict)"(reference=w1021) -> ("Value"=w1020:T1)  [unwired: 1 in, 2 out]
            n364 = Unbundle By Name(w1020) -> ("Bottom Position"=w1019:dbl)
            n365 = Unbundle By Name(w1015) -> ("Main Clean Cart"=w1016:refnum<vi>)
            n366 = property class="Bool (strict)"(reference=w1030, "Value"=FALSE) -> ()  [unwired: 1 in, 2 out]
            n367 = property class="Bool (strict)"(reference=w1016, "Value"=FALSE, "DisabledEnum"=T13."Enabled" ("Disabled")) -> ()  [unwired: 1 in, 2 out]
            n368 = call "Zaber Manager.vi"("Action"=Mot_Stage_Mngr."Abs Move", "Value"=w1019, "error in (no error)"=w1032) -> ("error out"=w1013:errorcluster)  [unwired: 6 in, 6 out]
            n369 = call "DAQ Manager.vi"("DAQ Mngr Action"=DAQ_Mngr."Pinch Valve Disengage", "error in (no error)"=w1013) -> ("error out"=w1012:errorcluster)  [unwired: 7 in, 6 out]
            n370 = call "Update Cart Status.vi"("Selection"=status_update."Cartridge", "error in (no error)"=w1012, "String"="Finished", "Array"=w1033, "FP"=w1015) -> ("error out"=w1025:errorcluster)  [unwired: 6 in]
            n371 = call "Update Cart Status.vi"("Selection"=status_update."Main Status", "error in (no error)"=w1025, "String"="Thermal Wash is finished, please remove catridges" ("Current Status"), "FP"=w1015) -> ("error out"=w1024:errorcluster)  [unwired: 7 in]
          }
          frame "-rinse wells" {
            n372 = call "Update Cart Status.vi"("Selection"=status_update."Main Status", "error in (no error)"=w1050, "String"="Draining All Wells and Lines", "FP"=w1043) -> ("error out"=w1049:errorcluster)  [unwired: 7 in]
            n373 = Unbundle By Name(w1043) -> ("Config"=w1056:refnum<vi>)
            n374 = property class="Clust (strict)"(reference=w1056) -> ("Value"=w1055:T1)  [unwired: 1 in, 2 out]
            n375 = Unbundle By Name(w1055) -> ("Load Position"=w1054:dbl)
            n376 = call "Zaber Manager.vi"("Action"=Mot_Stage_Mngr."Abs Move", "Value"=w1054, "error in (no error)"=w1049) -> ("error out"=w1053:errorcluster)  [unwired: 6 in, 6 out]
            n377 = call "Run Script.vi"("Script Name"="Drain All Wells", "Main References"=w1043, "error in (no error)"=w1053) -> ("error out"=w1044:errorcluster)  [unwired: 8 in]
            n378 = for {
              N: w1045 -> [w1067]
              shift-right: [w1070] -> w1041
              shift-left: w1044 -> [w1066]
              tunnel: w1043 -> [w1064]
              tunnel: w1043 -> [w1063]
              i -> [w1069]
              n379 = Format Into String(format string="Rinse %d of %d", w1069, w1067) -> (resulting string=w1065:string)  [unwired: 2 in, 1 out]
              n380 = call "Update Cart Status.vi"("Selection"=status_update."Main Status", "error in (no error)"=w1066, "String"=w1065, "FP"=w1064) -> ("error out"=w1071:errorcluster)  [unwired: 7 in]
              n381 = call "Run Script.vi"("Script Name"="Rinse All Wells", "Main References"=w1063, "error in (no error)"=w1071) -> ("error out"=w1070:errorcluster)  [unwired: 8 in]
            }
            n382 = Select(t=Process_State."Error" ("State"), s=w1041, f=Process_State."Idle" ("State")) -> (s? t:f=w1060:T5)
          }
          frame "-fill well" {
            # "Move to TW position if we are not doing liquid check"
            n383 = Unbundle By Name(w1086) -> ("Commands"=w1085:refnum<vi>)
            n384 = property class="Clust (strict)"(reference=w1085) -> ("Value"=w1084:T29)  [unwired: 1 in, 2 out]
            n385 = Unbundle By Name(w1084) -> ("Well #"=w1076:T30, "Bottle #"=w1077:T18)
            n386 = Format Into String(format string="Filling %s with %s", w1076, w1077) -> (resulting string=w1078:string)  [unwired: 2 in, 1 out]
            n387 = call "Update Cart Status.vi"("Selection"=status_update."Main Status", "error in (no error)"=w1083, "String"=w1078, "FP"=w1086) -> ("error out"=w1081:errorcluster)  [unwired: 7 in]
            n388 = call "Run Script.vi"("Script Name"="Fill Well_X Reagent_X" ("name or relative path"), "Main References"=w1086, "error in (no error)"=w1081, "Well X"=w1076, "Bottle X"=w1077) -> ("error out"=w1075:errorcluster)  [unwired: 6 in]
            n389 = Select(t=Process_State."PrePresTest" ("State"), s=w1094, f=Process_State."Idle" ("State")) -> (s? t:f=w1092:T5)
            n390 = Select(t=Process_State."Error" ("State"), s=w1075, f=w1092) -> (s? t:f=w1091:T5)
          }
          frame "-drain all" {
            # "Move to TW position if we are not doing liquid check"
            n391 = Unbundle By Name(w1109) -> ("Commands"=w1108:refnum<vi>)
            n392 = property class="Clust (strict)"(reference=w1108) -> ("Value"=w1107:T29)  [unwired: 1 in, 2 out]
            n393 = Unbundle By Name(w1107) -> ("Well #"=w1101:T30, "Bottle #"=w1102:T18)
            n394 = call "Update Cart Status.vi"("Selection"=status_update."Main Status", "error in (no error)"=w1106, "String"="Draining all wells" ("format string"), "FP"=w1109) -> ("error out"=w1104:errorcluster)  [unwired: 7 in]
            n395 = call "Run Script.vi"("Script Name"="Drain All Wells" ("name or relative path"), "Main References"=w1109, "error in (no error)"=w1104, "Well X"=w1101, "Bottle X"=w1102) -> ("error out"=w1100:errorcluster)  [unwired: 6 in]
            n396 = Select(t=Process_State."PrePresTest" ("State"), s=w1117, f=Process_State."Idle" ("State")) -> (s? t:f=w1115:T5)
            n397 = Select(t=Process_State."Error" ("State"), s=w1100, f=w1115) -> (s? t:f=w1114:T5)
          }
          frame "-clean cartridge" {
            # "clean time"
            # "TODO:  do all of this with one script\nneed to add Pressure X to script handler"
            n398 = call "Update Cart Status.vi"("Selection"=status_update."Main Status", "error in (no error)"=w1161, "String"="Cleaning cartridge", "FP"=w1122) -> ("error out"=w1141:errorcluster)  [unwired: 7 in]
            n399 = for {
              shift-right: [w1183] -> w1140
              shift-left: w1141 -> [w1184]
              tunnel: w1122 -> [w1182]
              tunnel: w1125 -> [w1181] mode=indexing
              tunnel: "Drain Well X" ("name or relative path") -> [w1180]
              i -> [w1179]
              n400 = case shown="True" w1181 {
                tunnel: w1184 -> [w1185 w1190]
                tunnel: [w1185 w1188] -> w1183
                tunnel: w1182 -> [_ w1189]
                tunnel: w1180 -> [_ w1187]
                tunnel: w1179 -> [_ w1186]
                frame False {
                }
                frame True {
                  n401 = call "Run Script.vi"("Script Name"=w1187, "Main References"=w1189, "error in (no error)"=w1190, "Drain X"=w1186, "Well X"=w1186) -> ("error out"=w1188:errorcluster)  [unwired: 6 in]
                }
              }
            }
            n402 = Unbundle By Name(w1122) -> ("Commands"=w1159:refnum<vi>)
            n403 = Unbundle By Name(w1122) -> ("Config"=w1149:refnum<vi>)
            n404 = for {
              shift-right: [w1170] -> w1138
              shift-left: w1140 -> [w1171]
              tunnel: w1122 -> [w1169]
              tunnel: w1125 -> [w1168] mode=indexing
              tunnel: "Fill Well_X Reagent_X" ("name or relative path") -> [w1167]
              i -> [w1166]
              n405 = case shown="True" w1168 {
                tunnel: w1171 -> [w1172 w1178]
                tunnel: [w1172 w1176] -> w1170
                tunnel: w1169 -> [_ w1177]
                tunnel: w1167 -> [_ w1175]
                tunnel: w1166 -> [_ w1174]
                frame False {
                }
                frame True {
                  n406 = call "Run Script.vi"("Script Name"=w1175, "Main References"=w1177, "error in (no error)"=w1178, "Drain X"=w1174, "Well X"=w1174, "Bottle X"=Bottles."H2O") -> ("error out"=w1176:errorcluster)  [unwired: 5 in]
                }
              }
            }
            n407 = property class="Clust (strict)"(reference=w1149) -> ("Value"=w1148:T1)  [unwired: 1 in, 2 out]
            n408 = Unbundle By Name(w1148) -> ("Load Position"=w1147:dbl, "TW Position"=w1132:dbl, "Dry Time(s)"=w1128:dbl)
            n409 = property class="Clust (strict)"(reference=w1159) -> (reference out=w1153:refnum<vi>, "Value"=w1155:T29)  [unwired: 1 in, 1 out]
            n410 = call "Zaber Manager.vi"("Action"=Mot_Stage_Mngr."Abs Move", "Value"=w1132, "error in (no error)"=w1138) -> ("error out"=w1136:errorcluster)  [unwired: 6 in, 6 out]
            n411 = call "Denkovi Manager.vi"("Action"=Denkovi_Mngr."Pres ON", "error in (no error)"=w1136, "Relays In"=w1125) -> ("error out"=w1133:errorcluster)  [unwired: 6 in, 2 out]
            n412 = call "Delay with Cancel 2.vi"("Insert Error"=FALSE, "error in (no error)"=w1133, "Delay(s)"=180.0) -> ("error out"=w1131:errorcluster)  [unwired: 7 in, 1 out]
            n413 = Bundle By Name(cluster=w1155, "Clean&Dry Cartridge"=FALSE ("Check for leaks")) -> (w1152:T29)
            n414 = call "Zaber Manager.vi"("Action"=Mot_Stage_Mngr."Abs Move", "Value"=w1147, "error in (no error)"=w1131) -> ("error out"=w1129:errorcluster)  [unwired: 6 in, 6 out]
            n415 = call "Delay with Cancel 2.vi"("Insert Error"=FALSE, "error in (no error)"=w1129, "Delay(s)"=w1128) -> ("error out"=w1126:errorcluster)  [unwired: 7 in, 1 out]
            n416 = call "Denkovi Manager.vi"("Action"=Denkovi_Mngr."Vent&Close", "error in (no error)"=w1126, "Relays In"=w1125) -> ("error out"=w1124:errorcluster)  [unwired: 6 in, 2 out]
            n417 = for {
              shift-right: [w1195] -> w1146
              shift-left: w1124 -> [w1196]
              tunnel: w1122 -> [w1194]
              tunnel: w1125 -> [w1193] mode=indexing
              tunnel: "Drain Well X" ("name or relative path") -> [w1192]
              i -> [w1191]
              n418 = case shown="True" w1193 {
                tunnel: w1196 -> [w1197 w1202]
                tunnel: [w1197 w1200] -> w1195
                tunnel: w1194 -> [_ w1201]
                tunnel: w1192 -> [_ w1199]
                tunnel: w1191 -> [_ w1198]
                frame False {
                }
                frame True {
                  n419 = call "Run Script.vi"("Script Name"=w1199, "Main References"=w1201, "error in (no error)"=w1202, "Drain X"=w1198, "Well X"=w1198) -> ("error out"=w1200:errorcluster)  [unwired: 6 in]
                }
              }
            }
            n420 = property class="Clust (strict)"(reference=w1153, error in=w1146, "Value"=w1152) -> (error out=w1145:errorcluster)  [unwired: 1 out]
            n421 = Select(t=Process_State."Error" ("State"), s=w1145, f=Process_State."Idle" ("State")) -> (s? t:f=w1164:T5)
          }
          frame "-check cartridge" {
            n422 = call "Update Cart Status.vi"("Selection"=status_update."Main Status", "error in (no error)"=w1234, "String"="Checking cartridge", "FP"=w1221) -> ("error out"=w1208:errorcluster)  [unwired: 7 in]
            n423 = call "DAQ Manager.vi"("DAQ Mngr Action"=DAQ_Mngr."Pinch Valve Engage", "error in (no error)"=w1208) -> ("error out"=w1207:errorcluster)  [unwired: 7 in, 6 out]
            n424 = Unbundle By Name(w1221) -> ("Commands"=w1232:refnum<vi>)
            n425 = disable-structure shown="Enabled" {
              disable-tunnel: [w1258 w1273] -> w1228
              disable-tunnel: w1221 -> [w1257 _]
              disable-tunnel: w1211 -> [w1256 _]
              disable-tunnel: w1207 -> [w1255 w1273]
              frame Disabled {
                n426 = for {
                  shift-right: [w1262] -> w1258
                  shift-left: w1255 -> [w1263]
                  tunnel: w1257 -> [w1261]
                  tunnel: w1256 -> [w1260] mode=indexing
                  i -> [w1259]
                  n427 = case shown="True" w1260 {
                    tunnel: w1263 -> [w1264 w1270]
                    tunnel: [w1264 w1268] -> w1262
                    tunnel: w1261 -> [_ w1267]
                    tunnel: w1259 -> [_ w1265]
                    frame False {
                    }
                    frame True {
                      n428 = call "Run Script.vi"("Script Name"="Drain Well X" ("name or relative path"), "Main References"=w1267, "error in (no error)"=w1270, "Drain X"=w1265, "Well X"=w1265) -> ("error out"=w1269:errorcluster)  [unwired: 6 in]
                      n429 = call "Run Script.vi"("Script Name"="Fill Well_X Reagent_X" ("name or relative path"), "Main References"=w1267, "error in (no error)"=w1269, "Drain X"=w1265, "Well X"=w1265, "Bottle X"=Bottles."H2O") -> ("error out"=w1268:errorcluster)  [unwired: 5 in]
                    }
                  }
                }
              }
              frame Enabled {
              }
            }
            n430 = Unbundle By Name(w1221) -> ("Config"=w1220:refnum<vi>)
            n431 = property class="Clust (strict)"(reference=w1220) -> ("Value"=w1219:T1)  [unwired: 1 in, 2 out]
            n432 = property class="Clust (strict)"(reference=w1232) -> (reference out=w1225:refnum<vi>, "Value"=w1227:T29)  [unwired: 1 in, 1 out]
            n433 = Unbundle By Name(w1219) -> ("Bottom Position"=w1218:dbl)
            n434 = call "Detect Transition to TW.vi"("Main References"=w1221, "error in (no error)"=w1228, "Cart Array"=w1211) -> ("error out"=w1213:errorcluster, "Analysis"=w1214:T7[])  [unwired: 7 in]
            n435 = call "Denkovi Manager.vi"("Action"=Denkovi_Mngr."Vent&Close", "error in (no error)"=w1213, "Relays In"=w1211) -> ("error out"=w1212:errorcluster)  [unwired: 6 in, 2 out]
            n436 = Bundle By Name(cluster=w1227, "Check for leaks"=FALSE, "Cart Test Array"=w1214) -> (w1224:T29)
            n437 = call "Zaber Manager.vi"("Action"=Mot_Stage_Mngr."Abs Move", "Value"=w1218, "error in (no error)"=w1212) -> ("error out"=w1205:errorcluster)  [unwired: 6 in, 6 out]
            n438 = call "DAQ Manager.vi"("DAQ Mngr Action"=DAQ_Mngr."Pinch Valve Disengage", "error in (no error)"=w1205) -> ("error out"=w1204:errorcluster)  [unwired: 7 in, 6 out]
            n439 = disable-structure shown="Enabled" {
              disable-tunnel: w1204 -> [w1242 w1254]
              disable-tunnel: w1221 -> [w1241 _]
              disable-tunnel: [w1240 w1254] -> w1217
              disable-tunnel: w1211 -> [w1239 _]
              frame Disabled {
                n440 = for {
                  shift-right: [w1246] -> w1240
                  shift-left: w1242 -> [w1247]
                  tunnel: w1241 -> [w1245]
                  tunnel: w1239 -> [w1244] mode=indexing
                  i -> [w1243]
                  n441 = case shown="True" w1244 {
                    tunnel: w1247 -> [w1248 w1252]
                    tunnel: [w1248 w1250] -> w1246
                    tunnel: w1245 -> [_ w1251]
                    tunnel: w1243 -> [_ w1249]
                    frame False {
                    }
                    frame True {
                      n442 = call "Run Script.vi"("Script Name"="Drain Well X" ("name or relative path"), "Main References"=w1251, "error in (no error)"=w1252, "Drain X"=w1249, "Well X"=w1249) -> ("error out"=w1250:errorcluster)  [unwired: 6 in]
                    }
                  }
                }
              }
              frame Enabled {
              }
            }
            n443 = property class="Clust (strict)"(reference=w1225, error in=w1217, "Value"=w1224) -> (error out=w1216:errorcluster)  [unwired: 1 out]
            n444 = Select(t=Process_State."Error" ("State"), s=w1216, f=Process_State."Idle" ("State")) -> (s? t:f=w1237:T5)
          }
        }
      }
    }
    frame Error {
      (unwired) T31 {"negative limit switch"=FALSE, "positive limit switch"=FALSE, "home switch"=FALSE, "position marker"=FALSE, "device enable"=FALSE, "quick stop"=FALSE, "general purpose J"=FALSE, "general purpose I"=FALSE, "general purpose H"=FALSE, "general purpose G"=FALSE, "general purpose F"=FALSE, "general purpose E"=FALSE, "general purpose D"=FALSE, "general purpose C"=FALSE, "general purpose B"=FALSE, "general purpose A"=FALSE} ("digital inputs")
    }
  }
  "error out" <- w11
  "Wash Array" <- w6
  "State Out" <- w7
  "Reports" <- w4
